vi "mainui.vi"() -> ()   [LabVIEW 2011]
uses:
  <vilib>/Platform/TimedLoop/XDataNode/timing_clust.ctl
  <vilib>/Platform/TimedLoop/XDataNode/nitl_modes.ctl
  <vilib>/Platform/TimedLoop/XDataNode/wakeup.ctl
  <vilib>/Utility/config.llb/Read Key (Double).vi
  <vilib>/Utility/config.llb/Read Key (I32).vi
  <vilib>/Utility/config.llb/Read Key (String).vi
  <vilib>/Utility/config.llb/Write Key (Double).vi
  <vilib>/Utility/config.llb/Write Key (I32).vi
  <vilib>/Utility/config.llb/Write Key (String).vi
  <vilib>/Platform/TimedLoop/XDataNode/XDataNode.xnode
  API/API DYM.lvlib
  <vilib>/Platform/TimedLoop/XDataNode/XDNodeRunTimeDep.lvlib
  <vilib>/Utility/config.llb/NI_LVConfig.lvlib
panel:
  in  "选项卡控件Next":enum32{"选项卡 1", "选项卡 2"}(tab)
  in  "BaseBtn":bool
  in  "MotinAdv":bool
  in  "restartbtn":bool
  in  "No1Btn":bool
  in  "No2Btn":bool
  in  "No3Btn":bool
  in  "Sensor":bool
  in  "选项卡控件":T1(tab)
  in  "ClearButton":bool
  out "红外计数":dbl
  out "电涡流计数":dbl
  out "红外电平":dbl
  out "电涡流电平":dbl
  out "电容1":dbl
  out "电容2":dbl
  out "电容3":dbl
  out "电桥电平":dbl
  out "电桥称重":dbl
  out "Waveform Chart":dynamicdata(graph)
  out "M1":bool
  out "M2":bool
  out "M3":bool
  out "M4":bool
  out "M5":bool
  out "M6":bool
  out "Plat3IO1":bool
  out "Plat3IO2":bool
  out "Plat3IO3":bool
  out "Plat3IO4":bool
  out "Plat3IO5":bool
  out "Plat3IO6":bool
  out "Plat3IO7":bool
  out "Plat3IO8":bool
  out "Plat2IO1":bool
  out "Plat2IO2":bool
  out "Plat2IO3":bool
  out "Plat2IO4":bool
  out "Plat2IO5":bool
  out "Plat2IO6":bool
  out "Plat2IO7":bool
  out "Plat2IO8":bool
  out "Solen48":bool
  out "Solen47":bool
  out "Solen46":bool
  out "Solen45":bool
  out "Solen44":bool
  out "Solen43":bool
  out "Solen42":bool
  out "Solen41":bool
  out "Solen40":bool
  out "Solen39":bool
  out "Solen38":bool
  out "Solen37":bool
  out "Solen36":bool
  out "Solen35":bool
  out "Solen34":bool
  out "Solen33":bool
  out "Solen32":bool
  out "Solen31":bool
  out "Solen30":bool
  out "Solen29":bool
  out "Solen28":bool
  out "Solen27":bool
  out "Solen26":bool
  out "Solen25":bool
  out "Solen24":bool
  out "Solen23":bool
  out "Solen22":bool
  out "Solen21":bool
  out "Solen20":bool
  out "Solen19":bool
  out "Solen18":bool
  out "Solen17":bool
  out "Solen16":bool
  out "Solen15":bool
  out "Solen14":bool
  out "Solen13":bool
  out "Solen12":bool
  out "Solen11":bool
  out "Solen10":bool
  out "Solen9":bool
  out "Solen8":bool
  out "Solen7":bool
  out "Solen6":bool
  out "Solen5":bool
  out "Solen4":bool
  out "Solen3":bool
  out "Solen2":bool
  out "Solen1":bool
  out "Plat1IO1":bool
  out "Plat1IO2":bool
  out "Plat1IO3":bool
  out "Plat1IO4":bool
  out "Plat1IO5":bool
  out "Plat1IO6":bool
  out "Plat1IO7":bool
  out "Plat1IO8":bool
  in  "MinSpeed":i32
  in  "MaxSpeed":i32
  in  "Horizontal4":i32
  in  "Horizontal3":i32
  in  "Horizontal2":i32
  in  "Horizontal1":i32
  in  "Vax4":i32
  in  "Vax3":i32
  in  "Vax2":i32
  in  "Vax1":i32
  in  "SaveParam":bool
  in  "CalcKB":bool
  out "BCalcd":dbl
  out "KCalcd":dbl
  out "Stog":dbl
  in  "Set2":bool
  in  "Set1":bool
  out "电桥电平_Event":dbl
  out "Volt2":dbl
  out "Volt1":dbl
  in  "X2":dbl
  in  "X1":dbl
  out "BCurrent":dbl
  out "KCurrent":dbl
  in  "SelectPolicy":enum32{"使用最短路径算法", "使用最短时间算法", "使用默认速度算法"}(radio)
  in  "ComboPolicy":string(combo)
  in  "ShowImg":bool
  in  "SaveConfigXZ":bool
  in  "SetReset":bool
  in  "MotorSpeed":i32=1
  in  "MotorSpeedNum":i32=1 min=1 max=6 step=1
  in  "SetMotorSpeed":bool
  out "Motor6Pos":i32
  out "Motor5Pos":i32
  out "Motor4Pos":i32
  out "Motor3Pos":i32
  out "Motor2Pos":i32
  out "Motor1Pos":i32
  in  "ClearPos6":bool
  in  "ClearPos5":bool
  in  "ClearPos4":bool
  in  "ClearPos3":bool
  in  "ClearPos2":bool
  in  "ClearPos1":bool
  in  "StopMotorNum":i32=1 min=1 max=6 step=1
  in  "StepNum":i32=1 min=1 max=20000 step=1
  in  "Directon":string(combo)
  in  "MotorNum":i32=1 min=1 max=6 step=1
  in  "SolenPlatStatue_Event":string(combo)
  in  "SolenPlat_Event":i32 min=0 max=2 step=1
  in  "SolenStatue_Event":string(combo)
  in  "SolenNum_Event":i32 min=0 max=47 step=1
  in  "MotorStop":bool
  in  "MotorStart":bool
  in  "FeedMotorStop":bool
  in  "FeedMotorStart":bool
  in  "SolenAdvance":bool
  in  "SolenAction":bool
  out "指令数":i32
  out "Statue":bool
  in  "start":bool
  in  "stop":bool
  in  "statuebtn":bool
  in  "no3btn":bool
  in  "no2btn":bool
  in  "no1btn":bool
  # "连接状态"
  # "待执行指令"
  # "红外计数"
  # "电涡流计数"
  # "电桥物体称重"
  # "红外传感器电平"
  # "电涡流传感器电平"
  # "电容式传感器1电平"
  # "电容式传感器2电平"
  # "电容式传感器3电平"
  # "电桥传感器电平"
  # "继电器状态"
  # "输入口状态"
  # "电机运行状态"
  # "单台控制策略——点位控制"
  # "单台控制策略——书写控制"
  # "当前电桥传感器矫正参数"
  # "g"
  # "K值"
  # "B值"
  # "当前传感器电压"
  # "mv"
  # "当前转换重量"
  # "电桥传感器参数标定"
  # "K值"
  # "B值"
  # "g"
  # "砝码重量1"
  # "对应电压"
  # "mv"
  # "砝码重量2"
  # "对应电压"
  # "g"
  # "mv"
  # "立体仓库坐标参数"
  # "第一行定位坐标Z轴"
  # "第一列定位坐标X轴"
  # "第二行定位坐标Z轴"
  # "第二列定位坐标X轴"
  # "第三行定位坐标Z轴"
  # "第三列定位坐标X轴"
  # "第四行定位坐标Z轴"
  # "第四列定位坐标X轴"
  # "电机参数"
  # "放置策略"
  # "电机最大速度"
  # "电机最小速度"
  # "策略选择"
  # "脉冲/S"
  # "脉冲/S"
  # "电机联动算法"
  # "继电器状态"
  # "继电器编号"
  # "继电器状态"
  # "平台编号"
  # "(进料电机运行)"
  # "电机速度"
  # "电机编号"
  # "脉冲/S"
  # "(进料电机停止)"
  # "电机编号"
  # "方向"
  # "步数"
  # "(1-20000)"
  # "电机编号"
  # "1号电机位置值:"
  # "4号电机位置值:"
  # "2号电机位置值:"
  # "5号电机位置值:"
  # "3号电机位置值:"
  # "6号电机位置值:"
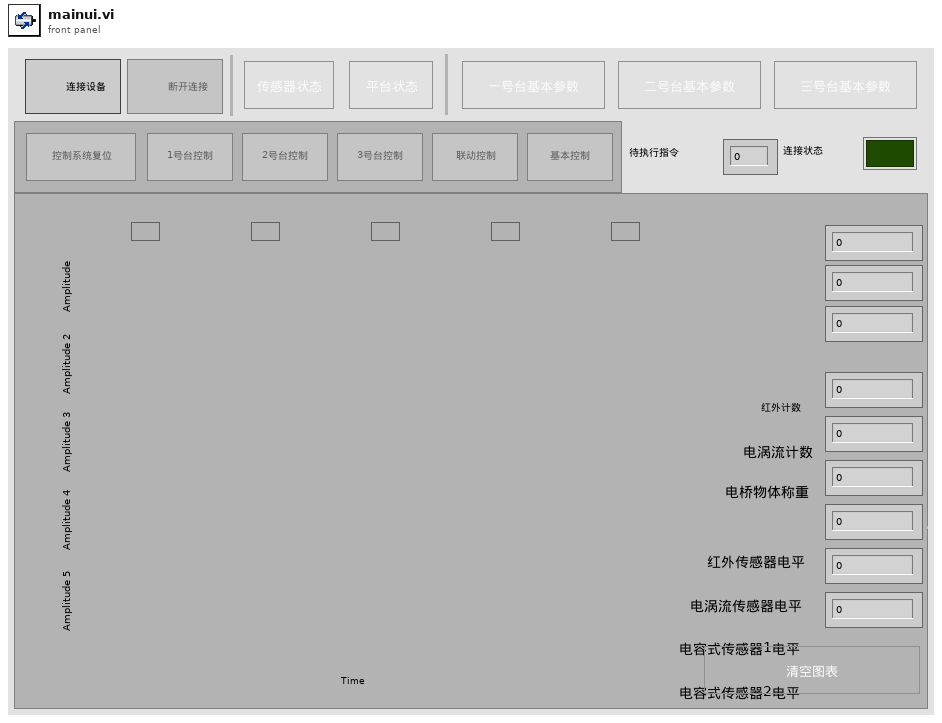
[diagram p1: front panel]
types:
  T1 = enum32{"选项卡 1", "选项卡 2", "选项卡 3", "选项卡 4", "选项卡 5", "选项卡 6"}
  T2 = enum8{"Enabled", "Disabled", "Disabled and Grayed Out"}
  T3 = enum16{"None", "GetSensorStatue", "GetSensorAD", "GetSolenStatue", "GetPaltformStatue", "GetMotorStatue", "FeedMotorStart", "FeedMotorStop", "MotorStart", "MotorRestart", "MotorStop", "SolenAction", "SolenAdv", "RcvDataInit", "SetMotorSpeed"}
  T4 = typedef "NI_LVConfig.lvlib/Config Data RefNum.ctl" = refnum<k1>
  T5 = enum16{"None", "GetSensorStatue", "GetSensorAD", "GetSolenStatue", "GetPaltformStatue", "GetMotorStatue", "FeedMotorStart", "FeedMotorStop", "MotorStart", "MotorRestart", "MotorStop", "SolenAction", "SolenAdv", "RcvDataInit"}
  T6 = typedef "XDNodeRunTimeDep.lvlib/timing_clust.ctl" = cluster{"Expected End [f-1]":u64, "Actual End [f-1]":u64, "Finished Late? [f-1]":bool, "Expected End [i-1]":u64, "Actual End [i-1]":u64, "Finished Late? [i-1]":bool, "Expected Start [i]":u64, "Actual Start [i]":u64, "Expected Start [f]":u64, "Actual Start [f]":u64, "Source Name":string, "Structure Name":string, "Period":i64, "Deadline":i64, "Offset":i64, "Start":i64, "Priority":i32, "Timeout":i32, "Mode":T7, "Wakeup Reason":T8, "Error":errorcluster, "Source Type":string, "Secondary Source Type":string, "Global End Time":u64, "Global Start Time":u64, "Frame Duration":u64, "Iteration Duration":u64, "Assigned CPU":i32, "I/O Scan Engine Mode":u32}
  T7 = typedef "XDNodeRunTimeDep.lvlib/nitl_modes.ctl" = enum32{"No Change", "Process missed periods, maintain original phase", "Discard missed periods, maintain original phase", "Process missed periods, ignore original phase", "Discard missed periods, ignore original phase"}
  T8 = typedef "XDNodeRunTimeDep.lvlib/wakeup.ctl" = enum32{"Normal", "Aborted", "Asynchronous wakeup", "Timing source error", "Timed loop error", "Timeout"}
  T9 = enum16{"None", "GetSensorStatue", "GetSensorAD", "GetSolenStatue", "GetPaltformStatue", "GetMotorStatue", "FeedMotorStart", "FeedMotorStop", "MotorStart", "MotorRestart", "MotorStop", "SolenAction", "SolenAdv"}
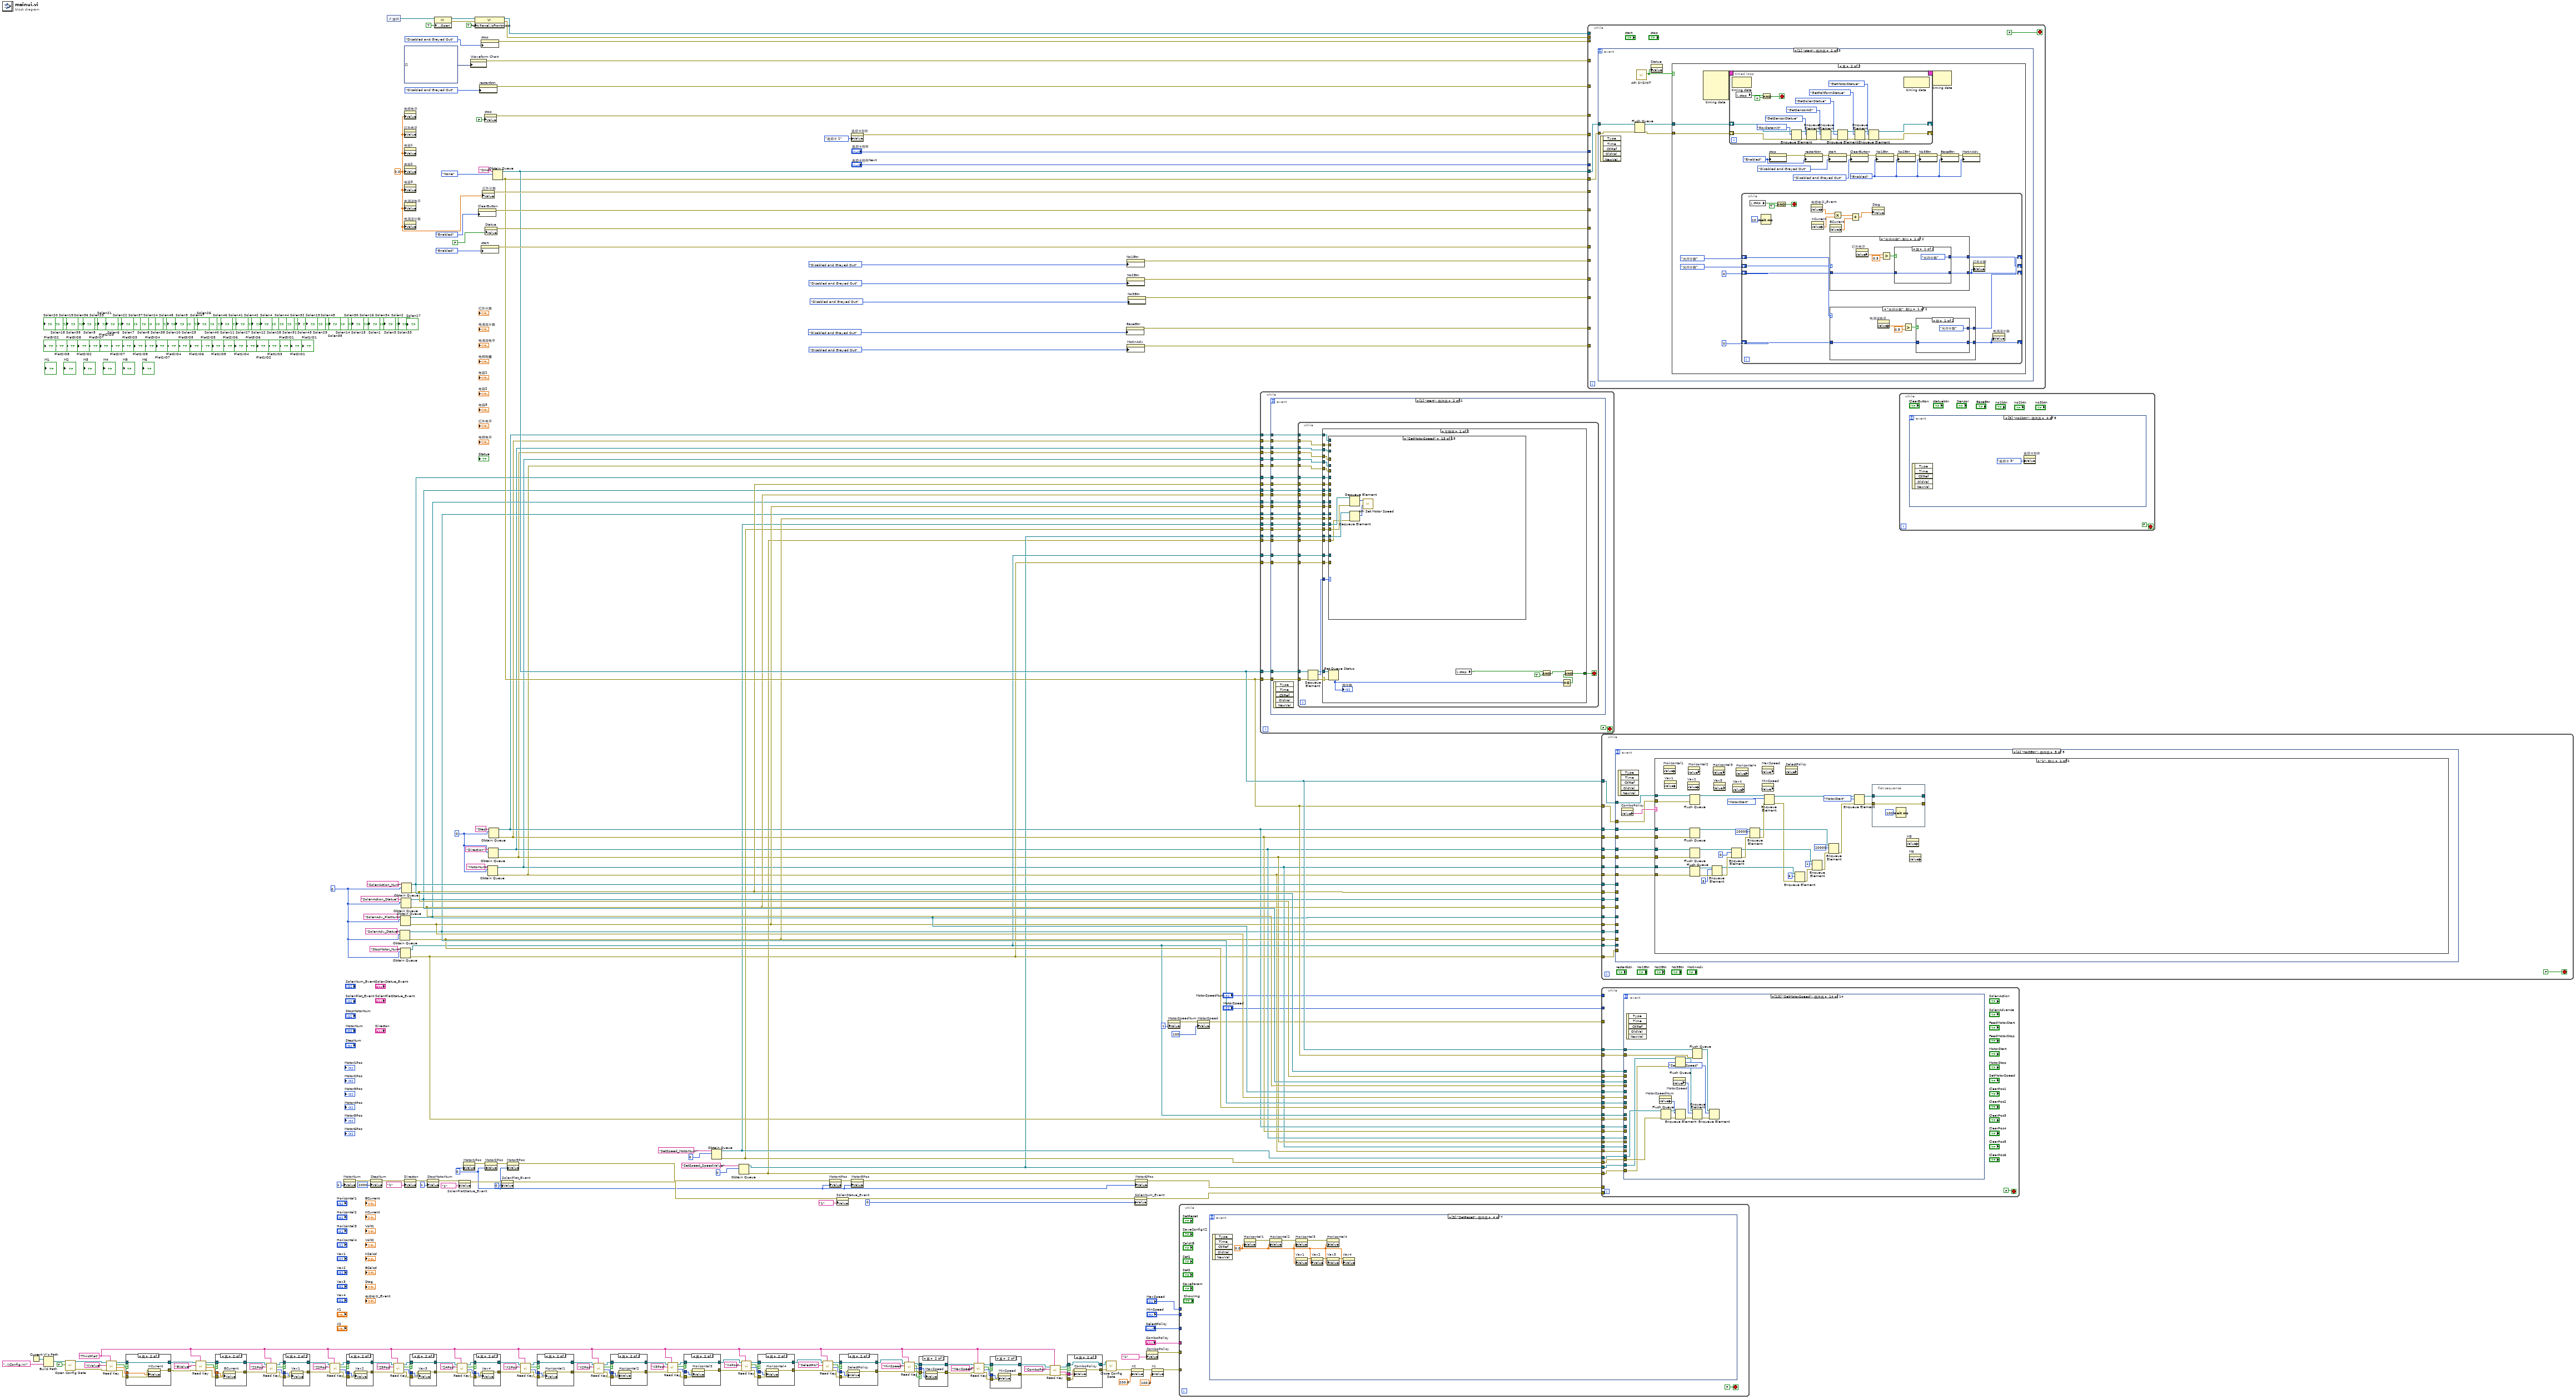
[diagram p0: block diagram]
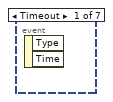
[diagram p16: hidden frame]
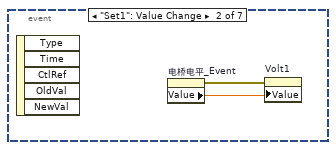
[diagram p17: hidden frame]
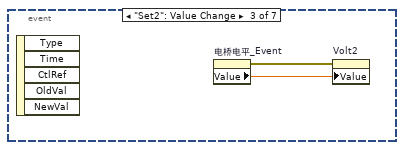
[diagram p18: hidden frame]
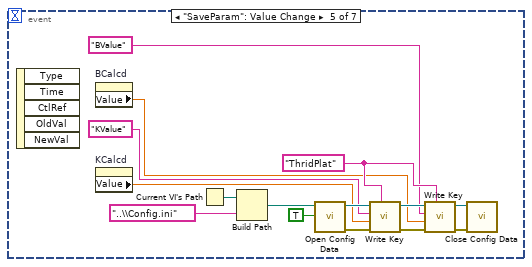
[diagram p19: hidden frame]
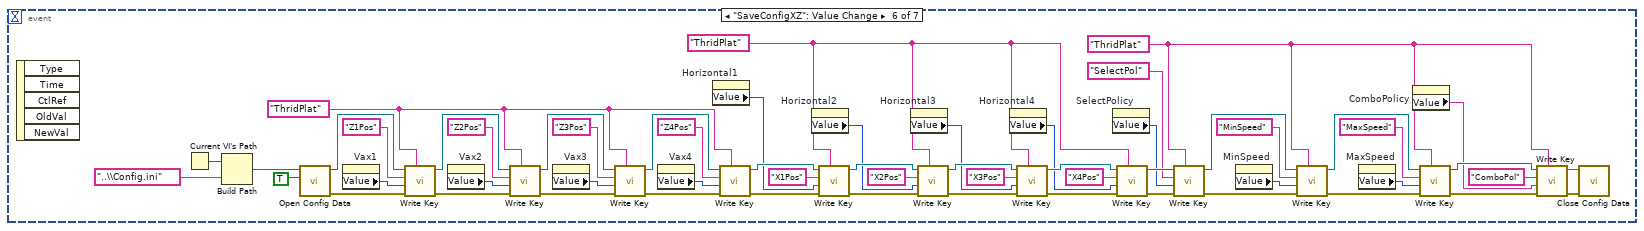
[diagram p20: hidden frame]
diagram:
  w2 = "ThridPlat" ("section")
  w135 = 0 ("Motor1Pos")
  w157 = 0
  w192 = 0
  w211 = 0.0
  n1 = Current VI's Path() -> (path=w129:path)
  n2 = Build Path(base path=w129, name or relative path="..\\Config.ini" ("名称或相对路径")) -> (appended path=w127:path)
  n3 = call <vilib>:"Open Config Data.vi"("create file if necessary (T)"=TRUE, "configuration file path"=w127) -> ("error out"=w124:errorcluster, "refnum"=w125:T4)  [unwired: 7 in, 1 out]
  n4 = call-poly <vilib>:"Read Key.vi"("section"=w2, "error in (no error)"=w124, "key"="KValue", "refnum"=w125) -> ("error out"=w120:errorcluster, "value"=w121:dbl, "found?"=w122:bool, "refnum out"=w119:T4)  [unwired: 4 in]
  n5 = case shown="真" w122 {
    tunnel: w121 -> [_ w226]
    tunnel: w120 -> [w221 w225]
    tunnel: [w221 w224] -> w117
    tunnel: [w222 w223] -> w118
    tunnel: w119 -> [w222 w223]
    frame False {
    }
    frame True {
      n6 = property on="KCurrent" class="DigNum (严格)"(error in=w225, "Value"=w226) -> (error out=w224:errorcluster)  [unwired: 1 in, 1 out]
    }
  }
  n7 = call-poly <vilib>:"Read Key.vi"("section"=w2, "error in (no error)"=w117, "key"="BValue", "refnum"=w118) -> ("error out"=w113:errorcluster, "value"=w112:dbl, "found?"=w115:bool, "refnum out"=w114:T4)  [unwired: 4 in]
  n8 = case shown="真" w115 {
    tunnel: [w228 w232] -> w111
    tunnel: w114 -> [w228 w232]
    tunnel: w113 -> [w227 w231]
    tunnel: [w227 w230] -> w110
    tunnel: w112 -> [_ w229]
    frame False {
    }
    frame True {
      n9 = property on="BCurrent" class="DigNum (严格)"(error in=w231, "Value"=w229) -> (error out=w230:errorcluster)  [unwired: 1 in, 1 out]
    }
  }
  n10 = call-poly <vilib>:"Read Key.vi"("section"=w2, "error in (no error)"=w110, "key"="Z1Pos", "refnum"=w111) -> ("error out"=w106:errorcluster, "value"=w105:i32, "found?"=w108:bool, "refnum out"=w107:T4)  [unwired: 4 in]
  n11 = case shown="真" w108 {
    tunnel: [w234 w238] -> w104
    tunnel: w107 -> [w234 w238]
    tunnel: w106 -> [w233 w237]
    tunnel: [w233 w236] -> w103
    tunnel: w105 -> [_ w235]
    frame False {
    }
    frame True {
      n12 = property on="Vax1" class="DigNum (严格)"(error in=w237, "Value"=w235) -> (error out=w236:errorcluster)  [unwired: 1 in, 1 out]
    }
  }
  n13 = call-poly <vilib>:"Read Key.vi"("section"=w2, "error in (no error)"=w103, "key"="Z2Pos", "refnum"=w104) -> ("error out"=w99:errorcluster, "value"=w98:i32, "found?"=w101:bool, "refnum out"=w100:T4)  [unwired: 4 in]
  n14 = property on="MotorNum" class="DigNum (严格)"("Value"=1 ("MotorNum")) -> (error out=w141:errorcluster)  [unwired: 2 in, 1 out]
  n15 = case shown="真" w101 {
    tunnel: w100 -> [w240 w244]
    tunnel: [w240 w244] -> w97
    tunnel: w99 -> [w239 w242]
    tunnel: w98 -> [_ w243]
    tunnel: [w239 w241] -> w96
    frame False {
    }
    frame True {
      n16 = property on="Vax2" class="DigNum (严格)"(error in=w242, "Value"=w243) -> (error out=w241:errorcluster)  [unwired: 1 in, 1 out]
    }
  }
  n17 = property on="StepNum" class="DigNum (严格)"(error in=w141, "Value"=2000 ("StepNum")) -> (error out=w144:errorcluster)  [unwired: 1 in, 1 out]
  n18 = control-ref of="本VI"() -> (w210:refnum<vi>)
  n19 = call-poly <vilib>:"Read Key.vi"("section"=w2, "error in (no error)"=w96, "key"="Z3Pos", "refnum"=w97) -> ("error out"=w92:errorcluster, "value"=w91:i32, "found?"=w94:bool, "refnum out"=w93:T4)  [unwired: 4 in]
  n20 = Obtain Queue(name (unnamed)="SolenAdv_Statue" ("名称（未命名）"), element data type=w157) -> (queue out=w160:refnum<queue>, error out=w159:errorcluster)  [unwired: 3 in, 1 out]
  n21 = Obtain Queue(name (unnamed)="SolenAdv_PlatNum" ("名称（未命名）"), element data type=w157) -> (queue out=w162:refnum<queue>, error out=w161:errorcluster)  [unwired: 3 in, 1 out]
  n22 = Obtain Queue(name (unnamed)="StopMotor_Num" ("名称（未命名）"), element data type=w157) -> (queue out=w156:refnum<queue>, error out=w155:errorcluster)  [unwired: 3 in, 1 out]
  n23 = Obtain Queue(name (unnamed)="SolenAction_Statue" ("名称（未命名）"), element data type=w157) -> (queue out=w168:refnum<queue>, error out=w167:errorcluster)  [unwired: 3 in, 1 out]
  n24 = Obtain Queue(name (unnamed)="SolenAction_Num" ("名称（未命名）"), element data type=w157) -> (queue out=w170:refnum<queue>, error out=w169:errorcluster)  [unwired: 3 in, 1 out]
  n25 = property on="电桥电平" class="DigNum (严格)"("Value"=w211) -> ()  [unwired: 2 in, 2 out]
  n26 = property on="红外电平" class="DigNum (严格)"("Value"=w211) -> ()  [unwired: 2 in, 2 out]
  n27 = property on="电容1" class="DigNum (严格)"("Value"=w211) -> ()  [unwired: 2 in, 2 out]
  n28 = property on="电容2" class="DigNum (严格)"("Value"=w211) -> ()  [unwired: 2 in, 2 out]
  n29 = property on="电容3" class="DigNum (严格)"("Value"=w211) -> ()  [unwired: 2 in, 2 out]
  n30 = property on="电涡流电平" class="DigNum (严格)"("Value"=w211) -> ()  [unwired: 2 in, 2 out]
  n31 = property on="电涡流计数" class="DigNum (严格)"("Value"=w211) -> ()  [unwired: 2 in, 2 out]
  n32 = property on="Directon" class="CmbBox"(error in=w144, "Value"="1" ("Directon")) -> (error out=w145:errorcluster)  [unwired: 1 in, 1 out]
  n33 = case shown="真" w94 {
    tunnel: w93 -> [w246 w250]
    tunnel: [w246 w250] -> w90
    tunnel: w92 -> [w245 w248]
    tunnel: w91 -> [_ w249]
    tunnel: [w245 w247] -> w89
    frame False {
    }
    frame True {
      n34 = property on="Vax3" class="DigNum (严格)"(error in=w248, "Value"=w249) -> (error out=w247:errorcluster)  [unwired: 1 in, 1 out]
    }
  }
  n35 = property on="StopMotorNum" class="DigNum (严格)"(error in=w145, "Value"=1 ("StopMotorNum")) -> (error out=w147:errorcluster)  [unwired: 1 in, 1 out]
  n36 = property class="VI"(reference=w210, "Front Panel.Open"=TRUE ("前面板窗口:打开")) -> (reference out=w208:refnum<vi>, error out=w207:errorcluster)  [unwired: 1 in]
  n37 = call-poly <vilib>:"Read Key.vi"("section"=w2, "error in (no error)"=w89, "key"="Z4Pos", "refnum"=w90) -> ("error out"=w85:errorcluster, "value"=w84:i32, "found?"=w87:bool, "refnum out"=w86:T4)  [unwired: 4 in]
  n38 = property on="SolenPlatStatue_Event" class="CmbBox"(error in=w147, "Value"="1" ("SolenPlatStatue_Event")) -> (error out=w164:errorcluster)  [unwired: 1 in, 1 out]
  n39 = property on="Motor1Pos" class="DigNum (严格)"("Value"=w135) -> (error out=w139:errorcluster)  [unwired: 2 in, 1 out]
  n40 = property on="Waveform Chart" class="WFChart (严格)"("History Data"=dynamicdata[] [] ("历史数据")) -> (error out=w218:errorcluster)  [unwired: 2 in, 1 out]
  n41 = case shown="真" w87 {
    tunnel: w86 -> [w252 w256]
    tunnel: w85 -> [w251 w254]
    tunnel: [w252 w256] -> w83
    tunnel: w84 -> [_ w255]
    tunnel: [w251 w253] -> w82
    frame False {
    }
    frame True {
      n42 = property on="Vax4" class="DigNum (严格)"(error in=w254, "Value"=w255) -> (error out=w253:errorcluster)  [unwired: 1 in, 1 out]
    }
  }
  n43 = property class="VI"(reference=w208, error in=w207, "Front Panel.IsFrontmost"=TRUE ("前面板窗口:在最前")) -> (reference out=w206:refnum<vi>, error out=w205:errorcluster)
  n44 = property on="ClearButton" class="Bool (严格)"("DisabledEnum"=T2."Enabled" ("禁用")) -> (error out=w216:errorcluster)  [unwired: 2 in, 1 out]
  n45 = property on="restartbtn" class="Bool"("DisabledEnum"=T2."Disabled and Grayed Out" ("禁用")) -> (error out=w200:errorcluster)  [unwired: 2 in, 1 out]
  n46 = property on="stop" class="Bool (严格)"("DisabledEnum"=T2."Disabled and Grayed Out" ("禁用")) -> (error out=w214:errorcluster)  [unwired: 2 in, 1 out]
  n47 = property on="start" class="Bool"("DisabledEnum"=T2."Enabled" ("禁用")) -> (error out=w215:errorcluster)  [unwired: 2 in, 1 out]
  n48 = property on="红外计数" class="DigNum (严格)"("Value"=w211) -> (error out=w220:errorcluster)  [unwired: 2 in, 1 out]
  n49 = property on="stop" class="Bool (严格)"("Value"=FALSE ("stop")) -> (error out=w196:errorcluster)  [unwired: 2 in, 1 out]
  n50 = property on="Statue" class="Bool (严格)"("Value"=FALSE ("Statue")) -> (error out=w202:errorcluster)  [unwired: 2 in, 1 out]
  n51 = property on="Motor2Pos" class="DigNum (严格)"(error in=w139, "Value"=w135) -> (error out=w140:errorcluster)  [unwired: 1 in, 1 out]
  n52 = Obtain Queue(name (unnamed)="MotorNum" ("名称（未命名）"), element data type=w192) -> (queue out=w150:refnum<queue>, error out=w149:errorcluster)  [unwired: 3 in, 1 out]
  n53 = Obtain Queue(name (unnamed)="Direction" ("名称（未命名）"), element data type=w192) -> (queue out=w152:refnum<queue>, error out=w151:errorcluster)  [unwired: 3 in, 1 out]
  n54 = Obtain Queue(name (unnamed)="Step" ("名称（未命名）"), element data type=w192) -> (queue out=w154:refnum<queue>, error out=w153:errorcluster)  [unwired: 3 in, 1 out]
  n55 = Obtain Queue(name (unnamed)="Cmd" ("名称（未命名）"), element data type=T3."None") -> (queue out=w172:refnum<queue>, error out=w171:errorcluster)  [unwired: 3 in, 1 out]
  n56 = property on="SolenPlat_Event" class="DigNum (严格)"(error in=w164, "Value"=0 ("SolenPlat_Event")) -> (error out=w166:errorcluster)  [unwired: 1 in, 1 out]
  n57 = property on="Motor3Pos" class="DigNum (严格)"(error in=w140, "Value"=w135) -> (error out=w138:errorcluster)  [unwired: 1 in, 1 out]
  n58 = call-poly <vilib>:"Read Key.vi"("section"=w2, "error in (no error)"=w82, "key"="X1Pos", "refnum"=w83) -> ("error out"=w79:errorcluster, "value"=w78:i32, "found?"=w77:bool, "refnum out"=w80:T4)  [unwired: 4 in]
  n59 = case shown="真" w77 {
    tunnel: w80 -> [w258 w262]
    tunnel: w79 -> [w257 w260]
    tunnel: [w258 w262] -> w76
    tunnel: w78 -> [_ w261]
    tunnel: [w257 w259] -> w75
    frame False {
    }
    frame True {
      n60 = property on="Horizontal1" class="DigNum (严格)"(error in=w260, "Value"=w261) -> (error out=w259:errorcluster)  [unwired: 1 in, 1 out]
    }
  }
  n61 = call-poly <vilib>:"Read Key.vi"("section"=w2, "error in (no error)"=w75, "key"="X2Pos", "refnum"=w76) -> ("error out"=w69:errorcluster, "value"=w68:i32, "found?"=w71:bool, "refnum out"=w70:T4)  [unwired: 4 in]
  n62 = case shown="真" w71 {
    tunnel: w70 -> [w264 w265]
    tunnel: w69 -> [w263 w267]
    tunnel: w68 -> [_ w268]
    tunnel: [w263 w266] -> w58
    tunnel: [w264 w265] -> w59
    frame False {
    }
    frame True {
      n63 = property on="Horizontal2" class="DigNum (严格)"(error in=w267, "Value"=w268) -> (error out=w266:errorcluster)  [unwired: 1 in, 1 out]
    }
  }
  n64 = call-poly <vilib>:"Read Key.vi"("section"=w2, "error in (no error)"=w58, "key"="X3Pos", "refnum"=w59) -> ("error out"=w64:errorcluster, "value"=w65:i32, "found?"=w67:bool, "refnum out"=w66:T4)  [unwired: 4 in]
  n65 = case shown="真" w67 {
    tunnel: w66 -> [w270 w272]
    tunnel: w65 -> [_ w274]
    tunnel: w64 -> [w269 w273]
    tunnel: [w270 w272] -> w57
    tunnel: [w269 w271] -> w56
    frame False {
    }
    frame True {
      n66 = property on="Horizontal3" class="DigNum (严格)"(error in=w273, "Value"=w274) -> (error out=w271:errorcluster)  [unwired: 1 in, 1 out]
    }
  }
  n67 = Obtain Queue(name (unnamed)="SetSpeed_MotorNum" ("名称（未命名）"), element data type=0) -> (queue out=w38:refnum<queue>, error out=w37:errorcluster)  [unwired: 3 in, 1 out]
  n68 = Obtain Queue(name (unnamed)="SetSpeed_SpeedValue" ("名称（未命名）"), element data type=0) -> (queue out=w36:refnum<queue>, error out=w35:errorcluster)  [unwired: 3 in, 1 out]
  n69 = call-poly <vilib>:"Read Key.vi"("section"=w2, "error in (no error)"=w56, "key"="X4Pos", "refnum"=w57) -> ("error out"=w61:errorcluster, "value"=w60:i32, "found?"=w63:bool, "refnum out"=w62:T4)  [unwired: 4 in]
  n70 = case shown="真" w63 {
    tunnel: w62 -> [w276 w280]
    tunnel: w61 -> [w275 w279]
    tunnel: w60 -> [_ w277]
    tunnel: [w276 w280] -> w33
    tunnel: [w275 w278] -> w32
    frame False {
    }
    frame True {
      n71 = property on="Horizontal4" class="DigNum (严格)"(error in=w279, "Value"=w277) -> (error out=w278:errorcluster)  [unwired: 1 in, 1 out]
    }
  }
  n72 = call-poly <vilib>:"Read Key.vi"("section"=w2, "error in (no error)"=w32, "key"="SelectPol", "refnum"=w33) -> ("error out"=w28:errorcluster, "value"=w27:i32, "found?"=w30:bool, "refnum out"=w29:T4)  [unwired: 4 in]
  n73 = property on="Motor4Pos" class="DigNum (严格)"(error in=w138, "Value"=w135) -> (error out=w137:errorcluster)  [unwired: 1 in, 1 out]
  n74 = property on="SolenStatue_Event" class="CmbBox"(error in=w166, "Value"="1" ("SolenStatue_Event")) -> (error out=w174:errorcluster)  [unwired: 1 in, 1 out]
  n75 = case shown="真" w30 {
    tunnel: w29 -> [w282 w286]
    tunnel: w28 -> [w281 w284]
    tunnel: w27 -> [_ w285]
    tunnel: [w282 w286] -> w26
    tunnel: [w281 w283] -> w25
    frame False {
    }
    frame True {
      n76 = property on="SelectPolicy" class="RadioBtnsControl (严格)"(error in=w284, "Value"=w285) -> (error out=w283:errorcluster)  [unwired: 1 in, 1 out]
    }
  }
  n77 = property on="选项卡控件" class="TabCtl (严格)"("Value"=T1."选项卡 1" ("选项卡控件")) -> (error out=w187:errorcluster)  [unwired: 2 in, 1 out]
  n78 = property on="Motor5Pos" class="DigNum (严格)"(error in=w137, "Value"=w135) -> (error out=w136:errorcluster)  [unwired: 1 in, 1 out]
  n79 = call-poly <vilib>:"Read Key.vi"("section"=w2, "error in (no error)"=w25, "key"="MinSpeed", "refnum"=w26) -> ("error out"=w23:errorcluster, "value"=w21:i32, "found?"=w1:bool, "refnum out"=w24:T4)  [unwired: 4 in]
  n80 = case shown="真" w1 {
    tunnel: w24 -> [w288 w292]
    tunnel: [w288 w292] -> w20
    tunnel: w23 -> [w287 w290]
    tunnel: w21 -> [_ w291]
    tunnel: [w287 w289] -> w19
    frame False {
    }
    frame True {
      n81 = property on="MaxSpeed" class="DigNum (严格)"(error in=w290, "Value"=w291) -> (error out=w289:errorcluster)  [unwired: 1 in, 1 out]
    }
  }
  n82 = call-poly <vilib>:"Read Key.vi"("section"=w2, "error in (no error)"=w19, "key"="MaxSpeed", "refnum"=w20) -> ("error out"=w15:errorcluster, "value"=w14:i32, "found?"=w17:bool, "refnum out"=w16:T4)  [unwired: 4 in]
  n83 = case shown="真" w17 {
    tunnel: w16 -> [w294 w295]
    tunnel: w15 -> [w293 w298]
    tunnel: w14 -> [_ w297]
    tunnel: [w293 w296] -> w12
    tunnel: [w294 w295] -> w13
    frame False {
    }
    frame True {
      n84 = property on="MinSpeed" class="DigNum (严格)"(error in=w298, "Value"=w297) -> (error out=w296:errorcluster)  [unwired: 1 in, 1 out]
    }
  }
  n85 = call-poly <vilib>:"Read Key.vi"("section"=w2, "error in (no error)"=w12, "key"="ComboPol", "refnum"=w13) -> ("error out"=w9:errorcluster, "value"=w7:string, "found?"=w8:bool, "refnum out"=w10:T4)  [unwired: 4 in]
  n86 = case shown="真" w8 {
    tunnel: w10 -> [w300 w301]
    tunnel: w9 -> [w299 w303]
    tunnel: w7 -> [_ w304]
    tunnel: [w299 w302] -> w5
    tunnel: [w300 w301] -> w6
    frame False {
    }
    frame True {
      n87 = property on="ComboPolicy" class="CmbBox"(error in=w303, "Value"=w304) -> (error out=w302:errorcluster)  [unwired: 1 in, 1 out]
    }
  }
  n88 = call <vilib>:"Close Config Data.vi"("error in (no error)"=w5, "refnum"=w6) -> ("error out"=w55:errorcluster)  [unwired: 8 in, 1 out]
  n89 = property on="BaseBtn" class="Bool"("DisabledEnum"=T2."Disabled and Grayed Out" ("禁用")) -> (error out=w180:errorcluster)  [unwired: 2 in, 1 out]
  n90 = property on="No1Btn" class="Bool"("DisabledEnum"=T2."Disabled and Grayed Out" ("禁用")) -> (error out=w186:errorcluster)  [unwired: 2 in, 1 out]
  n91 = property on="No2Btn" class="Bool"("DisabledEnum"=T2."Disabled and Grayed Out" ("禁用")) -> (error out=w184:errorcluster)  [unwired: 2 in, 1 out]
  n92 = property on="MotinAdv" class="Bool"("DisabledEnum"=T2."Disabled and Grayed Out" ("禁用")) -> (error out=w178:errorcluster)  [unwired: 2 in, 1 out]
  n93 = property on="No3Btn" class="Bool"("DisabledEnum"=T2."Disabled and Grayed Out" ("禁用")) -> (error out=w183:errorcluster)  [unwired: 2 in, 1 out]
  n94 = property on="X2" class="DigNum (严格)"(error in=w55, "Value"=200.0 ("X2")) -> (error out=w130:errorcluster)  [unwired: 1 in, 1 out]
  n95 = property on="SolenNum_Event" class="DigNum (严格)"(error in=w174, "Value"=0 ("SolenNum_Event")) -> (error out=w176:errorcluster)  [unwired: 1 in, 1 out]
  n96 = property on="Motor6Pos" class="DigNum (严格)"(error in=w136, "Value"=w135) -> (error out=w134:errorcluster)  [unwired: 1 in, 1 out]
  n97 = property on="ComboPolicy" class="CmbBox"("Value"="1" ("ComboPolicy")) -> (error out=w34:errorcluster)  [unwired: 2 in, 1 out]
  n98 = property on="X1" class="DigNum (严格)"(error in=w130, "Value"=100.0 ("X1")) -> (error out=w132:errorcluster)  [unwired: 1 in, 1 out]
  n99 = property on="MotorSpeedNum" class="DigNum (严格)"("Value"=1 ("MotorSpeedNum")) -> (error out=w48:errorcluster)  [unwired: 2 in, 1 out]
  n100 = while {
    tunnel: w132 -> [_]
    tunnel: "SelectPolicy" -> [_]
    tunnel: "ComboPolicy" -> [_]
    tunnel: "MaxSpeed" -> [_]
    tunnel: "MinSpeed" -> [_]
    tunnel: w34 -> [_]
    stop <- FALSE stop-if-true
    n101 = event shown="[3] \"SetReset\": 值改变" {
      selector: _ -> [_ _ _ _ _ _ _]
      dyn-events: _ -> [_ _ _ _ _ _ _]
      timeout: _ -> [_ _ _ _ _ _ _]
      event Timeout {
        n102 = event-data() -> ()  [unwired: 1 in, 2 out]
      }
      event "Set1": Value Change {
        n103 = event-data() -> ()  [unwired: 1 in, 5 out]
        n104 = property on="电桥电平_Event" class="DigNum (严格)"() -> (error out=w306:errorcluster, "Value"=w307:dbl)  [unwired: 2 in, 1 out]
        n105 = property on="Volt1" class="DigNum (严格)"(error in=w306, "Value"=w307) -> ()  [unwired: 1 in, 2 out]
      }
      event "Set2": Value Change {
        n106 = event-data() -> ()  [unwired: 1 in, 5 out]
        n107 = property on="电桥电平_Event" class="DigNum (严格)"() -> (error out=w309:errorcluster, "Value"=w308:dbl)  [unwired: 2 in, 1 out]
        n108 = property on="Volt2" class="DigNum (严格)"(error in=w309, "Value"=w308) -> ()  [unwired: 1 in, 2 out]
      }
      event "SetReset": Value Change {
        w310 = 0.0 ("Horizontal1")
        n109 = event-data() -> ()  [unwired: 1 in, 5 out]
        n110 = property on="Horizontal1" class="DigNum (严格)"("Value"=w310) -> (error out=w316:errorcluster)  [unwired: 2 in, 1 out]
        n111 = property on="Horizontal2" class="DigNum (严格)"(error in=w316, "Value"=w310) -> (error out=w315:errorcluster)  [unwired: 1 in, 1 out]
        n112 = property on="Horizontal3" class="DigNum (严格)"(error in=w315, "Value"=w310) -> (error out=w314:errorcluster)  [unwired: 1 in, 1 out]
        n113 = property on="Vax1" class="DigNum (严格)"("Value"=w310) -> (error out=w313:errorcluster)  [unwired: 2 in, 1 out]
        n114 = property on="Vax2" class="DigNum (严格)"(error in=w313, "Value"=w310) -> (error out=w312:errorcluster)  [unwired: 1 in, 1 out]
        n115 = property on="Horizontal4" class="DigNum (严格)"(error in=w314, "Value"=w310) -> ()  [unwired: 1 in, 2 out]
        n116 = property on="Vax3" class="DigNum (严格)"(error in=w312, "Value"=w310) -> (error out=w311:errorcluster)  [unwired: 1 in, 1 out]
        n117 = property on="Vax4" class="DigNum (严格)"(error in=w311, "Value"=w310) -> ()  [unwired: 1 in, 2 out]
      }
      event "SaveParam": Value Change {
        w323 = "ThridPlat" ("section")
        n118 = event-data() -> ()  [unwired: 1 in, 5 out]
        n119 = property on="BCalcd" class="DigNum (严格)"() -> ("Value"=w319:dbl)  [unwired: 2 in, 2 out]
        n120 = property on="KCalcd" class="DigNum (严格)"() -> ("Value"=w320:dbl)  [unwired: 2 in, 2 out]
        n121 = Current VI's Path() -> (path=w331:path)
        n122 = Build Path(base path=w331, name or relative path="..\\Config.ini" ("名称或相对路径")) -> (appended path=w329:path)
        n123 = call <vilib>:"Open Config Data.vi"("create file if necessary (T)"=TRUE, "configuration file path"=w329) -> ("error out"=w326:errorcluster, "refnum"=w327:T4)  [unwired: 7 in, 1 out]
        n124 = call-poly <vilib>:"Write Key.vi"("section"=w323, "error in (no error)"=w326, "value"=w320, "key"="KValue", "refnum"=w327) -> ("error out"=w324:errorcluster, "refnum out"=w325:T4)  [unwired: 4 in, 1 out]
        n125 = call-poly <vilib>:"Write Key.vi"("section"=w323, "error in (no error)"=w324, "value"=w319, "key"="BValue", "refnum"=w325) -> ("error out"=w317:errorcluster, "refnum out"=w318:T4)  [unwired: 4 in, 1 out]
        n126 = call <vilib>:"Close Config Data.vi"("error in (no error)"=w317, "refnum"=w318) -> ()  [unwired: 8 in, 2 out]
      }
      event "SaveConfigXZ": Value Change {
        w340 = "ThridPlat" ("section")
        w369 = "ThridPlat" ("section")
        w370 = "ThridPlat" ("section")
        n127 = event-data() -> ()  [unwired: 1 in, 5 out]
        n128 = Current VI's Path() -> (path=w388:path)
        n129 = Build Path(base path=w388, name or relative path="..\\Config.ini" ("名称或相对路径")) -> (appended path=w386:path)
        n130 = call <vilib>:"Open Config Data.vi"("create file if necessary (T)"=TRUE, "configuration file path"=w386) -> ("error out"=w365:errorcluster, "refnum"=w384:T4)  [unwired: 7 in, 1 out]
        n131 = property on="Vax1" class="DigNum (严格)"() -> ("Value"=w382:i32)  [unwired: 2 in, 2 out]
        n132 = call-poly <vilib>:"Write Key.vi"("section"=w370, "error in (no error)"=w365, "value"=w382, "key"="Z1Pos", "refnum"=w384) -> ("error out"=w378:errorcluster, "refnum out"=w381:T4)  [unwired: 4 in, 1 out]
        n133 = property on="Vax2" class="DigNum (严格)"() -> ("Value"=w358:i32)  [unwired: 2 in, 2 out]
        n134 = call-poly <vilib>:"Write Key.vi"("section"=w370, "error in (no error)"=w378, "value"=w358, "key"="Z2Pos", "refnum"=w381) -> ("error out"=w377:errorcluster, "refnum out"=w380:T4)  [unwired: 4 in, 1 out]
        n135 = property on="Vax3" class="DigNum (严格)"() -> ("Value"=w357:i32)  [unwired: 2 in, 2 out]
        n136 = call-poly <vilib>:"Write Key.vi"("section"=w370, "error in (no error)"=w377, "value"=w357, "key"="Z3Pos", "refnum"=w380) -> ("error out"=w376:errorcluster, "refnum out"=w379:T4)  [unwired: 4 in, 1 out]
        n137 = property on="Vax4" class="DigNum (严格)"() -> ("Value"=w355:i32)  [unwired: 2 in, 2 out]
        n138 = property on="Horizontal1" class="DigNum (严格)"() -> ("Value"=w354:i32)  [unwired: 2 in, 2 out]
        n139 = call-poly <vilib>:"Write Key.vi"("section"=w370, "error in (no error)"=w376, "value"=w355, "key"="Z4Pos", "refnum"=w379) -> ("error out"=w371:errorcluster, "refnum out"=w372:T4)  [unwired: 4 in, 1 out]
        n140 = property on="Horizontal2" class="DigNum (严格)"() -> ("Value"=w353:i32)  [unwired: 2 in, 2 out]
        n141 = call-poly <vilib>:"Write Key.vi"("section"=w369, "error in (no error)"=w371, "value"=w354, "key"="X1Pos", "refnum"=w372) -> ("error out"=w373:errorcluster, "refnum out"=w368:T4)  [unwired: 4 in, 1 out]
        n142 = property on="Horizontal3" class="DigNum (严格)"() -> ("Value"=w352:i32)  [unwired: 2 in, 2 out]
        n143 = call-poly <vilib>:"Write Key.vi"("section"=w369, "error in (no error)"=w373, "value"=w353, "key"="X2Pos", "refnum"=w368) -> ("error out"=w374:errorcluster, "refnum out"=w367:T4)  [unwired: 4 in, 1 out]
        n144 = property on="Horizontal4" class="DigNum (严格)"() -> ("Value"=w351:i32)  [unwired: 2 in, 2 out]
        n145 = call-poly <vilib>:"Write Key.vi"("section"=w369, "error in (no error)"=w374, "value"=w352, "key"="X3Pos", "refnum"=w367) -> ("error out"=w375:errorcluster, "refnum out"=w366:T4)  [unwired: 4 in, 1 out]
        n146 = property on="SelectPolicy" class="RadioBtnsControl (严格)"() -> ("Value"=w335:enum32{"使用最短路径算法", "使用最短时间算法", "使用默认速度算法"})  [unwired: 2 in, 2 out]
        n147 = call-poly <vilib>:"Write Key.vi"("section"=w369, "error in (no error)"=w375, "value"=w351, "key"="X4Pos", "refnum"=w366) -> ("error out"=w349:errorcluster, "refnum out"=w350:T4)  [unwired: 4 in, 1 out]
        n148 = call-poly <vilib>:"Write Key.vi"("section"=w340, "error in (no error)"=w349, "value"=w335, "key"="SelectPol", "refnum"=w350) -> ("error out"=w347:errorcluster, "refnum out"=w348:T4)  [unwired: 4 in, 1 out]
        n149 = property on="MinSpeed" class="DigNum (严格)"() -> ("Value"=w334:i32)  [unwired: 2 in, 2 out]
        n150 = call-poly <vilib>:"Write Key.vi"("section"=w340, "error in (no error)"=w347, "value"=w334, "key"="MinSpeed", "refnum"=w348) -> ("error out"=w345:errorcluster, "refnum out"=w346:T4)  [unwired: 4 in, 1 out]
        n151 = property on="MaxSpeed" class="DigNum (严格)"() -> ("Value"=w333:i32)  [unwired: 2 in, 2 out]
        n152 = property on="ComboPolicy" class="CmbBox"() -> ("Value"=w332:string)  [unwired: 2 in, 2 out]
        n153 = call-poly <vilib>:"Write Key.vi"("section"=w340, "error in (no error)"=w345, "value"=w333, "key"="MaxSpeed", "refnum"=w346) -> ("error out"=w343:errorcluster, "refnum out"=w344:T4)  [unwired: 4 in, 1 out]
        n154 = call-poly <vilib>:"Write Key.vi"("section"=w340, "error in (no error)"=w343, "value"=w332, "key"="ComboPol", "refnum"=w344) -> ("error out"=w341:errorcluster, "refnum out"=w342:T4)  [unwired: 4 in, 1 out]
        n155 = call <vilib>:"Close Config Data.vi"("error in (no error)"=w341, "refnum"=w342) -> ()  [unwired: 8 in, 2 out]
      }
      event "CalcKB": Value Change {
        n156 = event-data() -> ()  [unwired: 1 in, 5 out]
        n157 = property on="Volt1" class="DigNum (严格)"() -> ("Value"=w390:dbl)  [unwired: 2 in, 2 out]
        n158 = property on="Volt2" class="DigNum (严格)"() -> ("Value"=w389:dbl)  [unwired: 2 in, 2 out]
        n159 = Not Equal?(x=w390, y=w389) -> (x != y?=w391:bool)
        n160 = case shown="假" w391 {
          tunnel: w390 -> [_ w401]
          tunnel: w389 -> [_ w396]
          frame False {
            n161 = One Button Dialog(message="计算发生错误 !" ("消息")) -> ()  [unwired: 1 in, 1 out]
          }
          frame True {
            n162 = property on="X2" class="DigNum (严格)"() -> ("Value"=w394:dbl)  [unwired: 2 in, 2 out]
            n163 = property on="X1" class="DigNum (严格)"() -> ("Value"=w400:dbl)  [unwired: 2 in, 2 out]
            n164 = Subtract(x=w401, y=w396) -> (x-y=w398:dbl)
            n165 = Subtract(x=w400, y=w394) -> (x-y=w399:dbl)
            n166 = Divide(x=w399, y=w398) -> (x/y=w397:dbl)
            n167 = Multiply(x=w397, y=w396) -> (x*y=w395:dbl)
            n168 = Subtract(x=w394, y=w395) -> (x-y=w393:dbl)
            n169 = property on="KCalcd" class="DigNum (严格)"("Value"=w397) -> ()  [unwired: 2 in, 2 out]
            n170 = property on="BCalcd" class="DigNum (严格)"("Value"=w393) -> ()  [unwired: 2 in, 2 out]
          }
        }
      }
    }
  }
  n171 = property on="MotorSpeed" class="DigNum (严格)"(error in=w48, "Value"=100 ("MotorSpeed")) -> (error out=w47:errorcluster)  [unwired: 1 in, 1 out]
  n172 = while {
    tunnel: w172 -> [w422]
    tunnel: w171 -> [w423]
    tunnel: w154 -> [w421]
    tunnel: w153 -> [w420]
    tunnel: w152 -> [w419]
    tunnel: w151 -> [w418]
    tunnel: w150 -> [w417]
    tunnel: w149 -> [w416]
    tunnel: w170 -> [w415]
    tunnel: w169 -> [w414]
    tunnel: w168 -> [w413]
    tunnel: w167 -> [w412]
    tunnel: w162 -> [w411]
    tunnel: w161 -> [w410]
    tunnel: w160 -> [w409]
    tunnel: w159 -> [w408]
    tunnel: w156 -> [w407]
    tunnel: w155 -> [w406]
    tunnel: w38 -> [w405]
    tunnel: w37 -> [w404]
    tunnel: w36 -> [w403]
    tunnel: w35 -> [w402]
    stop <- FALSE stop-if-true
    n173 = event shown="[1] \"start\": 值改变" {
      selector: _ -> [_ _]
      dyn-events: _ -> [_ _]
      timeout: _ -> [_ _]
      tunnel: w423 -> [_ w446]
      tunnel: w422 -> [_ w445]
      tunnel: w421 -> [_ w444]
      tunnel: w420 -> [_ w443]
      tunnel: w419 -> [_ w442]
      tunnel: w418 -> [_ w441]
      tunnel: w417 -> [_ w440]
      tunnel: w416 -> [_ w439]
      tunnel: w415 -> [_ w438]
      tunnel: w414 -> [_ w437]
      tunnel: w413 -> [_ w436]
      tunnel: w412 -> [_ w435]
      tunnel: w411 -> [_ w434]
      tunnel: w410 -> [_ w433]
      tunnel: w409 -> [_ w432]
      tunnel: w408 -> [_ w431]
      tunnel: w407 -> [_ w430]
      tunnel: w406 -> [_ w429]
      tunnel: w405 -> [_ w428]
      tunnel: w404 -> [_ w427]
      tunnel: w403 -> [_ w426]
      tunnel: w402 -> [_ w425]
      event Timeout {
        n174 = event-data() -> ()  [unwired: 1 in, 2 out]
      }
      event "start": Value Change {
        n175 = event-data() -> ()  [unwired: 1 in, 5 out]
        n176 = while {
          tunnel: w446 -> [w467]
          tunnel: w445 -> [w468]
          tunnel: w444 -> [w462]
          tunnel: w443 -> [w461]
          tunnel: w442 -> [w464]
          tunnel: w441 -> [w463]
          tunnel: w440 -> [w466]
          tunnel: w439 -> [w465]
          tunnel: w438 -> [w460]
          tunnel: w437 -> [w459]
          tunnel: w436 -> [w458]
          tunnel: w435 -> [w457]
          tunnel: w434 -> [w456]
          tunnel: w433 -> [w455]
          tunnel: w432 -> [w454]
          tunnel: w431 -> [w453]
          tunnel: w430 -> [w452]
          tunnel: w429 -> [w451]
          tunnel: w428 -> [w450]
          tunnel: w427 -> [w449]
          tunnel: w426 -> [w448]
          tunnel: w425 -> [w447]
          stop <- w471 stop-if-true
          n177 = Dequeue Element(queue=w468, error in (no error)=w467) -> (queue out=w469:refnum<queue>, element=w472:T3, error out=w470:errorcluster)  [unwired: 1 in, 1 out]
          n178 = case shown="无错误" w470 {
            selector: w470 -> [w499 _]
            tunnel: w472 -> [w501 _]
            tunnel: [w479 TRUE] -> w471
            tunnel: w469 -> [w500 _]
            tunnel: w466 -> [w496 _]
            tunnel: w465 -> [w495 _]
            tunnel: w464 -> [w494 _]
            tunnel: w463 -> [w493 _]
            tunnel: w462 -> [w492 _]
            tunnel: w461 -> [w491 _]
            tunnel: w460 -> [w490 _]
            tunnel: w459 -> [w489 _]
            tunnel: w458 -> [w488 _]
            tunnel: w457 -> [w487 _]
            tunnel: w456 -> [w486 _]
            tunnel: w455 -> [w485 _]
            tunnel: w454 -> [w484 _]
            tunnel: w453 -> [w483 _]
            tunnel: w452 -> [w478 _]
            tunnel: w451 -> [w477 _]
            tunnel: w450 -> [w476 _]
            tunnel: w449 -> [w474 _]
            tunnel: w448 -> [w475 _]
            tunnel: w447 -> [w473 _]
            frame No Error {
              n179 = case shown="\"SetMotorSpeed\"" w501 {
                tunnel: w496 -> [_ _ _ _ _ _ _ _ w594 _ _ _ _ _ _]
                tunnel: w495 -> [_ _ _ _ _ _ _ _ w593 _ _ _ _ _ _]
                tunnel: w494 -> [_ _ _ _ _ _ _ _ w597 _ _ _ _ _ _]
                tunnel: w493 -> [_ _ _ _ _ _ _ _ w596 _ _ _ _ _ _]
                tunnel: w492 -> [_ _ _ _ _ _ _ _ w600 _ _ _ _ _ _]
                tunnel: w491 -> [_ _ _ _ _ _ _ _ w599 _ _ _ _ _ _]
                tunnel: w490 -> [_ _ _ _ _ _ _ _ _ _ _ w606 _ _ _]
                tunnel: w489 -> [_ _ _ _ _ _ _ _ _ _ _ w605 _ _ _]
                tunnel: w488 -> [_ _ _ _ _ _ _ _ _ _ _ w604 _ _ _]
                tunnel: w487 -> [_ _ _ _ _ _ _ _ _ _ _ w603 _ _ _]
                tunnel: w486 -> [_ _ _ _ _ _ _ _ _ _ _ _ w612 _ _]
                tunnel: w485 -> [_ _ _ _ _ _ _ _ _ _ _ _ w611 _ _]
                tunnel: w484 -> [_ _ _ _ _ _ _ _ _ _ _ _ w610 _ _]
                tunnel: w483 -> [_ _ _ _ _ _ _ _ _ _ _ _ w609 _ _]
                tunnel: w478 -> [_ _ _ _ _ _ _ _ _ _ _ _ _ _ _]
                tunnel: w477 -> [_ _ _ _ _ _ _ _ _ _ _ _ _ _ _]
                tunnel: w476 -> [_ _ _ _ _ _ _ _ _ _ _ _ _ _ w618]
                tunnel: w475 -> [_ _ _ _ _ _ _ _ _ _ _ _ _ _ w616]
                tunnel: w474 -> [_ _ _ _ _ _ _ _ _ _ _ _ _ _ w617]
                tunnel: w473 -> [_ _ _ _ _ _ _ _ _ _ _ _ _ _ w615]
                frame "None", Default {
                }
                frame "GetSensorStatue" {
                  n180 = Initialize Array(0 ("元素"), 8 ("维数大小")) -> (w504:i32[])
                  n181 = call "API get Sensor Statue.vi"("array input"=w504) -> ("array output"=w510:i32[])  [unwired: 9 in, 1 out]
                  n182 = Index Array(array=w510, index=2 ("索引")) -> (element=w518:i32)
                  n183 = Index Array(array=w510, index=1 ("索引")) -> (element=w517:i32)
                  n184 = Index Array(array=w510, index=4 ("索引")) -> (element=w519:i32)
                  n185 = Index Array(array=w510, index=5 ("索引")) -> (element=w520:i32)
                  n186 = Index Array(array=w510, index=3 ("索引")) -> (element=w521:i32)
                  n187 = property on="红外电平" class="DigNum (严格)"("Value"=w518) -> ()  [unwired: 2 in, 2 out]
                  n188 = property on="电涡流电平" class="DigNum (严格)"("Value"=w517) -> ()  [unwired: 2 in, 2 out]
                  n189 = property on="电容1" class="DigNum (严格)"("Value"=w519) -> ()  [unwired: 2 in, 2 out]
                  n190 = property on="电容2" class="DigNum (严格)"("Value"=w520) -> ()  [unwired: 2 in, 2 out]
                  n191 = property on="电容3" class="DigNum (严格)"("Value"=w521) -> ()  [unwired: 2 in, 2 out]
                  n192 = Merge Signals(w518) -> (w515:dynamicdata)
                  n193 = Merge Signals(w517) -> (w516:dynamicdata)
                  n194 = Merge Signals(w519) -> (w511:dynamicdata)
                  n195 = Merge Signals(w520) -> (w513:dynamicdata)
                  n196 = Merge Signals(w521) -> (w512:dynamicdata)
                  n197 = Merge Signals(w515, w516, w511, w513, w512) -> (→"Waveform Chart":dynamicdata)
                }
                frame "GetSensorAD" {
                  n198 = call "API get Sensor AD.vi"("SensorADValueIN"=0.0) -> ("SensorADValueOut"=w522:dbl)  [unwired: 3 in, 1 out]
                  n199 = property on="电桥电平" class="DigNum (严格)"("Value"=w522) -> ()  [unwired: 2 in, 2 out]
                  n200 = property on="电桥电平_Event" class="DigNum (严格)"("Value"=w522) -> ()  [unwired: 2 in, 2 out]
                }
                frame "GetSolenStatue" {
                  n201 = Initialize Array(0 ("元素"), 48 ("维数大小")) -> (w525:i32[])
                  n202 = call "API get solen statue.vi"("solenstatue input"=w525) -> ("solenstatue output"=w524:i32[])  [unwired: 10 in]
                  n203 = for {
                    tunnel: w524 -> [w531] mode=indexing
                    i -> [w534]
                    n204 = Not Equal To 0?(x=w531) -> (x != 0?=w532:bool)
                    n205 = Increment(x=w534) -> (x+1=w536:i32)
                    n206 = Number To Decimal String(number=w536) -> (decimal integer string=w535:string)  [unwired: 1 in]
                    n207 = To Variant(anything=w532) -> (Variant=w529:variant)
                    n208 = control-ref of="本VI"() -> (w530:refnum<vi>)
                    n209 = Concatenate Strings("Solen" ("字符串"), w535) -> (w528:string)
                    n210 = invoke class="VI" method="Ctrl Val.Set"(reference=w530, "Control Name"=w528, "Value"=w529) -> ()  [unwired: 2 in, 5 out]
                  }
                }
                frame "GetPaltformStatue" {
                  n211 = Initialize Array(0 ("元素"), 8 ("维数大小")) -> (w548:i32[])
                  n212 = Initialize Array(0 ("元素"), 8 ("维数大小")) -> (w545:i32[])
                  n213 = Initialize Array(0 ("元素"), 8 ("维数大小")) -> (w543:i32[])
                  n214 = call "API get platform statue.vi"("platformStatue input"=w548, "PlatformNum"=1) -> ("platformStatue output"=w537:i32[])  [unwired: 8 in, 1 out]
                  n215 = for {
                    tunnel: w537 -> [w555] mode=indexing
                    i -> [w558]
                    n216 = Not Equal To 0?(x=w555) -> (x != 0?=w556:bool)
                    n217 = To Variant(anything=w556) -> (Variant=w553:variant)
                    n218 = Increment(x=w558) -> (x+1=w560:i32)
                    n219 = Number To Decimal String(number=w560) -> (decimal integer string=w559:string)  [unwired: 1 in]
                    n220 = control-ref of="本VI"() -> (w554:refnum<vi>)
                    n221 = Concatenate Strings("Plat1IO" ("字符串"), w559) -> (w552:string)
                    n222 = invoke class="VI" method="Ctrl Val.Set"(reference=w554, "Control Name"=w552, "Value"=w553) -> ()  [unwired: 2 in, 5 out]
                  }
                  n223 = call "API get platform statue.vi"("platformStatue input"=w545, "PlatformNum"=3) -> ("platformStatue output"=w539:i32[])  [unwired: 8 in, 1 out]
                  n224 = call "API get platform statue.vi"("platformStatue input"=w543, "PlatformNum"=2) -> ("platformStatue output"=w538:i32[])  [unwired: 8 in, 1 out]
                  n225 = for {
                    tunnel: w539 -> [w573] mode=indexing
                    i -> [w576]
                    n226 = Increment(x=w576) -> (x+1=w578:i32)
                    n227 = Not Equal To 0?(x=w573) -> (x != 0?=w574:bool)
                    n228 = Number To Decimal String(number=w578) -> (decimal integer string=w577:string)  [unwired: 1 in]
                    n229 = control-ref of="本VI"() -> (w572:refnum<vi>)
                    n230 = Concatenate Strings("Plat3IO" ("字符串"), w577) -> (w570:string)
                    n231 = To Variant(anything=w574) -> (Variant=w571:variant)
                    n232 = invoke class="VI" method="Ctrl Val.Set"(reference=w572, "Control Name"=w570, "Value"=w571) -> ()  [unwired: 2 in, 5 out]
                  }
                  n233 = for {
                    tunnel: w538 -> [w564] mode=indexing
                    i -> [w567]
                    n234 = Increment(x=w567) -> (x+1=w569:i32)
                    n235 = Not Equal To 0?(x=w564) -> (x != 0?=w565:bool)
                    n236 = Number To Decimal String(number=w569) -> (decimal integer string=w568:string)  [unwired: 1 in]
                    n237 = control-ref of="本VI"() -> (w563:refnum<vi>)
                    n238 = Concatenate Strings("Plat2IO" ("字符串"), w568) -> (w561:string)
                    n239 = To Variant(anything=w565) -> (Variant=w562:variant)
                    n240 = invoke class="VI" method="Ctrl Val.Set"(reference=w563, "Control Name"=w561, "Value"=w562) -> ()  [unwired: 2 in, 5 out]
                  }
                }
                frame "GetMotorStatue" {
                  n241 = Initialize Array(0 ("元素"), 6 ("维数大小")) -> (w582:i32[])
                  n242 = call "API get motor statue.vi"("motor statue array input"=w582) -> ("motor statue array output"=w579:i32[])  [unwired: 9 in, 1 out]
                  n243 = for {
                    tunnel: w579 -> [w586] mode=indexing
                    i -> [w589]
                    n244 = Not Equal To 0?(x=w586) -> (x != 0?=w587:bool)
                    n245 = Increment(x=w589) -> (x+1=w591:i32)
                    n246 = Number To Decimal String(number=w591) -> (decimal integer string=w590:string)  [unwired: 1 in]
                    n247 = To Variant(anything=w587) -> (Variant=w584:variant)
                    n248 = control-ref of="本VI"() -> (w585:refnum<vi>)
                    n249 = Concatenate Strings("M" ("字符串"), w590) -> (w583:string)
                    n250 = invoke class="VI" method="Ctrl Val.Set"(reference=w585, "Control Name"=w583, "Value"=w584) -> ()  [unwired: 2 in, 5 out]
                  }
                }
                frame "FeedMotorStart" {
                  n251 = call "API Feed Motor START.vi"() -> ()  [unwired: 11 in, 1 out]
                }
                frame "FeedMotorStop" {
                  n252 = call "API Feed Motor Stop.vi"() -> ()  [unwired: 11 in, 1 out]
                }
                frame "MotorStart" {
                  n253 = Dequeue Element(queue=w594, error in (no error)=w593) -> (element=w592:i32)  [unwired: 1 in, 3 out]
                  n254 = Dequeue Element(queue=w600, error in (no error)=w599) -> (element=w598:i32)  [unwired: 1 in, 3 out]
                  n255 = Dequeue Element(queue=w597, error in (no error)=w596) -> (element=w595:i32)  [unwired: 1 in, 3 out]
                  n256 = call "API Motor Start.vi"("stepNum"=w598, "direction"=w595, "motorNum"=w592) -> ()  [unwired: 8 in, 1 out]
                }
                frame "MotorRestart" {
                }
                frame "MotorStop" {
                  n257 = call "API Motor Stop.vi"() -> ()  [unwired: 11 in, 1 out]
                }
                frame "SolenAction" {
                  n258 = Dequeue Element(queue=w604, error in (no error)=w603) -> (element=w601:i32)  [unwired: 1 in, 3 out]
                  n259 = Dequeue Element(queue=w606, error in (no error)=w605) -> (element=w602:i32)  [unwired: 1 in, 3 out]
                  n260 = call "API Solen Action.vi"("statue"=w601, "solenNum"=w602) -> ()  [unwired: 9 in, 1 out]
                }
                frame "SolenAdv" {
                  n261 = Dequeue Element(queue=w612, error in (no error)=w611) -> (element=w608:i32)  [unwired: 1 in, 3 out]
                  n262 = Dequeue Element(queue=w610, error in (no error)=w609) -> (element=w607:i32)  [unwired: 1 in, 3 out]
                  n263 = call "API Solen Advance.vi"("statue"=w607, "platformNum"=w608) -> ()  [unwired: 9 in, 1 out]
                }
                frame "RcvDataInit" {
                  n264 = call "API Rcv Data Init.vi"() -> ()  [unwired: 2 in, 2 out]
                }
                frame "SetMotorSpeed" {
                  n265 = Dequeue Element(queue=w618, error in (no error)=w617) -> (element=w614:i32)  [unwired: 1 in, 3 out]
                  n266 = Dequeue Element(queue=w616, error in (no error)=w615) -> (element=w613:i32)  [unwired: 1 in, 3 out]
                  n267 = call "API Set Motor Speed.vi"("motorSpeed"=w613, "motorNum"=w614) -> ()  [unwired: 9 in, 1 out]
                }
              }
              n268 = Get Queue Status(queue=w500, error in (no error)=w499) -> (# elements in queue=w482:i32)  [unwired: 1 in, 7 out]
              "指令数" <- w482
              n269 = local read "stop"() -> (w497:bool)
              n270 = And(x=w497, y=TRUE) -> (x .and. y?=w481:bool)
              n271 = Equal To 0?(x=w482) -> (x = 0?=w480:bool)
              n272 = And(x=w481, y=w480) -> (x .and. y?=w479:bool)
            }
            frame Error {
            }
          }
        }
      }
    }
  }
  n273 = while {
    tunnel: w220 -> [_]
    tunnel: w218 -> [_]
    tunnel: w216 -> [_]
    tunnel: w215 -> [_]
    tunnel: w214 -> [_]
    tunnel: w206 -> [_]
    tunnel: w205 -> [_]
    tunnel: w202 -> [_]
    tunnel: w200 -> [_]
    tunnel: w172 -> [w622]
    tunnel: w171 -> [w621]
    tunnel: w196 -> [_]
    tunnel: w187 -> [_]
    tunnel: w186 -> [_]
    tunnel: w184 -> [_]
    tunnel: w183 -> [_]
    tunnel: w180 -> [_]
    tunnel: w178 -> [_]
    tunnel: "选项卡控件" -> [_]
    tunnel: "选项卡控件Next" -> [_]
    stop <- FALSE stop-if-true
    n274 = event shown="[1] \"start\": 值改变" {
      selector: _ -> [_ _ _]
      dyn-events: _ -> [_ _ _]
      timeout: _ -> [_ _ _]
      tunnel: w622 -> [_ w626 w729]
      tunnel: w621 -> [_ w625 w728]
      event Timeout {
        n275 = event-data() -> ()  [unwired: 1 in, 2 out]
      }
      event "start": Value Change {
        n276 = event-data() -> ()  [unwired: 1 in, 5 out]
        n277 = Flush Queue(queue=w626, error in (no error)=w625) -> (queue out=w624:refnum<queue>, error out=w623:errorcluster)  [unwired: 1 out]
        n278 = call "API SYSINIT.vi"() -> ("SYSINIT return value"=w627:bool)  [unwired: 11 in]
        n279 = property on="Statue" class="Bool (严格)"("Value"=w627) -> ()  [unwired: 2 in, 2 out]
        n280 = case shown="真" w627 {
          tunnel: w624 -> [_ w637]
          tunnel: w623 -> [_ w636]
          frame False {
          }
          frame True {
            w630 = T2."Enabled" ("禁用")
            w641 = T2."Enabled" ("禁用")
            n281 = node-c288() -> (w629:T6)  [unwired: 4 in]
            n282 = timed-loop {
              shift-right: [w652] -> _
              shift-left: w637 -> [w660]
              shift-right: [w651] -> _
              shift-left: w636 -> [w659]
              timing: w629 -> [_]
              timing-out: [_] -> w628
              stop <- w648 stop-if-true
              n283 = node-c288() -> ()  [unwired: 1 in, 1 out]
              n284 = local read "stop"() -> (w649:bool)
              n285 = And(x=w649, y=TRUE) -> (x .and. y?=w648:bool)
              n286 = Enqueue Element(queue=w660, element=T5."RcvDataInit" ("元素"), error in (no error)=w659) -> (queue out=w662:refnum<queue>, error out=w661:errorcluster)  [unwired: 1 in, 1 out]
              n287 = Enqueue Element(queue=w662, element=T5."GetSensorStatue" ("元素"), error in (no error)=w661) -> (queue out=w670:refnum<queue>, error out=w669:errorcluster)  [unwired: 1 in, 1 out]
              n288 = Enqueue Element(queue=w670, element=T5."GetSensorAD" ("元素"), error in (no error)=w669) -> (queue out=w668:refnum<queue>, error out=w667:errorcluster)  [unwired: 1 in, 1 out]
              n289 = Enqueue Element(queue=w668, element=T5."GetSolenStatue" ("元素"), error in (no error)=w667) -> (queue out=w666:refnum<queue>, error out=w665:errorcluster)  [unwired: 1 in, 1 out]
              n290 = Enqueue Element(queue=w666, element=T5."GetPaltformStatue" ("元素"), error in (no error)=w665) -> (queue out=w664:refnum<queue>, error out=w663:errorcluster)  [unwired: 1 in, 1 out]
              n291 = Enqueue Element(queue=w664, element=T5."GetMotorStatue" ("元素"), error in (no error)=w663) -> (queue out=w652:refnum<queue>, error out=w651:errorcluster)  [unwired: 1 in, 1 out]
              n292 = node-c288() -> ()  [unwired: 1 in, 1 out]
            }
            n293 = while {
              shift-right: [w688] -> _
              shift-left: 0 -> [w690]
              shift-right: [w689] -> _
              shift-left: enum16{"允许计数", "不允许计数"}."允许计数" -> [w691]
              shift-right: [w682] -> _
              shift-left: enum16{"允许计数", "不允许计数"}."允许计数" -> [w684]
              shift-right: [w681] -> _
              shift-left: 0 -> [w683]
              stop <- w685 stop-if-true
              n294 = local read "stop"() -> (w687:bool)
              n295 = Wait (ms)(milliseconds to wait=u32 10 ("等待时间（毫秒）")) -> ()  [unwired: 1 out]
              n296 = And(x=w687, y=TRUE) -> (x .and. y?=w685:bool)
              n297 = property on="电桥电平_Event" class="DigNum (严格)"() -> ("Value"=w679:dbl)  [unwired: 2 in, 2 out]
              n298 = property on="KCurrent" class="DigNum (严格)"() -> ("Value"=w678:dbl)  [unwired: 2 in, 2 out]
              n299 = property on="BCurrent" class="DigNum (严格)"() -> ("Value"=w676:dbl)  [unwired: 2 in, 2 out]
              n300 = case shown="\"允许计数\", 默认" w684 {
                tunnel: w683 -> [w694 w703]
                tunnel: [w693 w703] -> w681
                tunnel: [w692 w704] -> w682
                frame "允许计数", Default {
                  n301 = property on="红外电平" class="DigNum (严格)"() -> ("Value"=w697:dbl)  [unwired: 2 in, 2 out]
                  n302 = Greater?(x=w697, y=0.5) -> (0:w695:bool)
                  n303 = case shown="假" w695 {
                    tunnel: w694 -> [w698 w702]
                    tunnel: [w698 w701] -> w693
                    tunnel: [enum16{"允许计数", "不允许计数"}."允许计数" enum16{"允许计数", "不允许计数"}."不允许计数"] -> w692
                    frame False {
                    }
                    frame True {
                      n304 = Increment(x=w702) -> (x+1=w701:i32)
                    }
                  }
                }
                frame "不允许计数" {
                  n305 = property on="红外电平" class="DigNum (严格)"() -> ("Value"=w707:dbl)  [unwired: 2 in, 2 out]
                  n306 = Less?(x=w707, y=0.5) -> (x < y?=w705:bool)
                  n307 = case shown="假" w705 {
                    tunnel: [enum16{"允许计数", "不允许计数"}."不允许计数" enum16{"允许计数", "不允许计数"}."允许计数"] -> w704
                    frame False {
                    }
                    frame True {
                    }
                  }
                }
              }
              n308 = case shown="\"允许计数\", 默认" w691 {
                tunnel: w690 -> [w712 w721]
                tunnel: [w711 w721] -> w688
                tunnel: [w710 w722] -> w689
                frame "允许计数", Default {
                  n309 = property on="电涡流电平" class="DigNum (严格)"() -> ("Value"=w715:dbl)  [unwired: 2 in, 2 out]
                  n310 = Greater?(x=w715, y=0.5) -> (0:w713:bool)
                  n311 = case shown="假" w713 {
                    tunnel: w712 -> [w716 w720]
                    tunnel: [w716 w719] -> w711
                    tunnel: [enum16{"允许计数", "不允许计数"}."允许计数" enum16{"允许计数", "不允许计数"}."不允许计数"] -> w710
                    frame False {
                    }
                    frame True {
                      n312 = Increment(x=w720) -> (x+1=w719:i32)
                    }
                  }
                }
                frame "不允许计数" {
                  n313 = property on="电涡流电平" class="DigNum (严格)"() -> ("Value"=w725:dbl)  [unwired: 2 in, 2 out]
                  n314 = Less?(x=w725, y=0.5) -> (x < y?=w723:bool)
                  n315 = case shown="假" w723 {
                    tunnel: [enum16{"允许计数", "不允许计数"}."不允许计数" enum16{"允许计数", "不允许计数"}."允许计数"] -> w722
                    frame False {
                    }
                    frame True {
                    }
                  }
                }
              }
              n316 = Multiply(x=w679, y=w678) -> (x*y=w677:dbl)
              n317 = Add(x=w677, y=w676) -> (x+y=w675:dbl)
              n318 = property on="Stog" class="DigNum (严格)"("Value"=w675) -> ()  [unwired: 2 in, 2 out]
              n319 = property on="红外计数" class="DigNum (严格)"("Value"=w681) -> ()  [unwired: 2 in, 2 out]
              n320 = property on="电涡流计数" class="DigNum (严格)"("Value"=w688) -> ()  [unwired: 2 in, 2 out]
            }
            n321 = property on="stop" class="Bool (严格)"("DisabledEnum"=w641) -> (error out=w640:errorcluster)  [unwired: 2 in, 1 out]
            n322 = property on="restartbtn" class="Bool"(error in=w640, "DisabledEnum"=w641) -> (error out=w639:errorcluster)  [unwired: 1 in, 1 out]
            n323 = property on="start" class="Bool"(error in=w639, "DisabledEnum"=T2."Disabled and Grayed Out" ("禁用")) -> (error out=w638:errorcluster)  [unwired: 1 in, 1 out]
            n324 = property on="ClearButton" class="Bool (严格)"(error in=w638, "DisabledEnum"=T2."Disabled and Grayed Out" ("禁用")) -> (error out=w635:errorcluster)  [unwired: 1 in, 1 out]
            n325 = property on="No1Btn" class="Bool"(error in=w635, "DisabledEnum"=w630) -> (error out=w634:errorcluster)  [unwired: 1 in, 1 out]
            n326 = property on="No2Btn" class="Bool"(error in=w634, "DisabledEnum"=w630) -> (error out=w633:errorcluster)  [unwired: 1 in, 1 out]
            n327 = property on="No3Btn" class="Bool"(error in=w633, "DisabledEnum"=w630) -> (error out=w632:errorcluster)  [unwired: 1 in, 1 out]
            n328 = node-c288(w628) -> ()  [unwired: 1 out]
            n329 = property on="BaseBtn" class="Bool"(error in=w632, "DisabledEnum"=w630) -> (error out=w631:errorcluster)  [unwired: 1 in, 1 out]
            n330 = property on="MotinAdv" class="Bool"(error in=w631, "DisabledEnum"=w630) -> ()  [unwired: 1 in, 2 out]
          }
        }
      }
      event "stop": Value Change {
        n331 = event-data() -> ()  [unwired: 1 in, 5 out]
        n332 = flat-sequence {
          tunnel: w729 -> [w731]
          tunnel: w728 -> [w730]
          frame #0 {
            n333 = Flush Queue(queue=w731, error in (no error)=w730) -> ()  [unwired: 3 out]
          }
          frame #1 {
            w732 = T2."Disabled and Grayed Out" ("禁用")
            n334 = property on="start" class="Bool"("DisabledEnum"=T2."Enabled" ("禁用")) -> (error out=w746:errorcluster)  [unwired: 2 in, 1 out]
            n335 = property on="stop" class="Bool (严格)"(error in=w746, "DisabledEnum"=T2."Disabled and Grayed Out" ("禁用")) -> (error out=w743:errorcluster)  [unwired: 1 in, 1 out]
            n336 = property on="stop" class="Bool (严格)"(error in=w743, "Value"=FALSE ("stop")) -> (error out=w742:errorcluster)  [unwired: 1 in, 1 out]
            n337 = property on="ClearButton" class="Bool (严格)"(error in=w742, "DisabledEnum"=T2."Enabled" ("禁用")) -> (error out=w740:errorcluster)  [unwired: 1 in, 1 out]
            n338 = property on="restartbtn" class="Bool"(error in=w740, "DisabledEnum"=w732) -> (error out=w739:errorcluster)  [unwired: 1 in, 1 out]
            n339 = property on="Statue" class="Bool (严格)"(error in=w739, "Value"=FALSE ("Statue")) -> (error out=w737:errorcluster)  [unwired: 1 in, 1 out]
            n340 = property on="No1Btn" class="Bool"(error in=w737, "DisabledEnum"=w732) -> (error out=w736:errorcluster)  [unwired: 1 in, 1 out]
            n341 = property on="No2Btn" class="Bool"(error in=w736, "DisabledEnum"=w732) -> (error out=w735:errorcluster)  [unwired: 1 in, 1 out]
            n342 = property on="No3Btn" class="Bool"(error in=w735, "DisabledEnum"=w732) -> (error out=w734:errorcluster)  [unwired: 1 in, 1 out]
            n343 = property on="BaseBtn" class="Bool"(error in=w734, "DisabledEnum"=w732) -> (error out=w733:errorcluster)  [unwired: 1 in, 1 out]
            n344 = property on="MotinAdv" class="Bool"(error in=w733, "DisabledEnum"=w732) -> ()  [unwired: 1 in, 2 out]
          }
          frame #2 {
            n345 = call "API SYSQUIT.vi"() -> ()  [unwired: 12 in]
          }
        }
      }
    }
  }
  n346 = while {
    tunnel: w171 -> [w764]
    tunnel: w172 -> [w765]
    tunnel: w154 -> [w763]
    tunnel: w153 -> [w762]
    tunnel: w152 -> [w761]
    tunnel: w151 -> [w760]
    tunnel: w150 -> [w759]
    tunnel: w149 -> [w758]
    tunnel: w170 -> [w757]
    tunnel: w168 -> [w756]
    tunnel: w162 -> [w755]
    tunnel: w160 -> [w754]
    tunnel: w169 -> [w753]
    tunnel: w167 -> [w752]
    tunnel: w161 -> [w751]
    tunnel: w159 -> [w750]
    tunnel: w156 -> [w749]
    tunnel: w155 -> [w748]
    stop <- FALSE stop-if-true
    n347 = event shown="[4] \"No3Btn\": 值改变" {
      selector: _ -> [_ _ _ _ _]
      dyn-events: _ -> [_ _ _ _ _]
      timeout: _ -> [_ _ _ _ _]
      tunnel: w765 -> [_ w808 w867 _ w924]
      tunnel: w764 -> [_ _ w866 _ w923]
      tunnel: w763 -> [_ w806 w865 _ w922]
      tunnel: w762 -> [_ w805 w864 _ w921]
      tunnel: w761 -> [_ w802 w863 _ w920]
      tunnel: w760 -> [_ _ w862 _ w919]
      tunnel: w759 -> [_ w801 w861 _ w918]
      tunnel: w758 -> [_ _ w860 _ w917]
      tunnel: w757 -> [_ _ w859 _ _]
      tunnel: w756 -> [_ _ w857 _ _]
      tunnel: w755 -> [_ w798 w855 _ _]
      tunnel: w754 -> [_ w797 w853 _ _]
      tunnel: w753 -> [_ _ w858 _ _]
      tunnel: w752 -> [_ _ w856 _ _]
      tunnel: w751 -> [_ _ w854 _ _]
      tunnel: w750 -> [_ _ w852 _ _]
      tunnel: w749 -> [_ _ _ _ _]
      tunnel: w748 -> [_ _ _ _ _]
      event Timeout {
        n348 = event-data() -> ()  [unwired: 1 in, 2 out]
      }
      event "restartbtn": Value Change {
        n349 = event-data() -> ()  [unwired: 1 in, 5 out]
        n350 = Flush Queue(queue=w806, error in (no error)=w805) -> (queue out=w804:refnum<queue>, error out=w803:errorcluster)  [unwired: 1 out]
        n351 = Enqueue Element(queue=w804, element=20000 ("元素"), error in (no error)=w803) -> (queue out=w844:refnum<queue>, error out=w850:errorcluster)  [unwired: 1 in, 1 out]
        n352 = Flush Queue(queue=w802) -> (queue out=w800:refnum<queue>)  [unwired: 1 in, 2 out]
        n353 = Enqueue Element(queue=w800, element=1 ("元素"), error in (no error)=w850) -> (queue out=w843:refnum<queue>, error out=w849:errorcluster)  [unwired: 1 in, 1 out]
        n354 = Flush Queue(queue=w801) -> (queue out=w799:refnum<queue>)  [unwired: 1 in, 2 out]
        n355 = Enqueue Element(queue=w799, element=3 ("元素"), error in (no error)=w849) -> (queue out=w842:refnum<queue>, error out=w848:errorcluster)  [unwired: 1 in, 1 out]
        n356 = Flush Queue(queue=w808) -> (queue out=w807:refnum<queue>)  [unwired: 1 in, 2 out]
        n357 = Enqueue Element(queue=w807, element=T9."MotorStart" ("元素"), error in (no error)=w848) -> (queue out=w837:refnum<queue>, error out=w841:errorcluster)  [unwired: 1 in, 1 out]
        n358 = Enqueue Element(queue=w844, element=20000 ("元素"), error in (no error)=w841) -> (queue out=w823:refnum<queue>, error out=w840:errorcluster)  [unwired: 1 in, 1 out]
        n359 = Enqueue Element(queue=w843, element=1 ("元素"), error in (no error)=w840) -> (queue out=w821:refnum<queue>, error out=w839:errorcluster)  [unwired: 1 in, 1 out]
        n360 = Enqueue Element(queue=w842, element=4 ("元素"), error in (no error)=w839) -> (queue out=w819:refnum<queue>, error out=w838:errorcluster)  [unwired: 1 in, 1 out]
        n361 = Enqueue Element(queue=w837, element=T9."MotorStart" ("元素"), error in (no error)=w838) -> (queue out=w829:refnum<queue>, error out=w832:errorcluster)  [unwired: 1 in, 1 out]
        n362 = Enqueue Element(queue=w823, element=20000 ("元素"), error in (no error)=w832) -> (queue out=w822:refnum<queue>, error out=w831:errorcluster)  [unwired: 1 in, 1 out]
        n363 = Enqueue Element(queue=w821, element=0 ("元素"), error in (no error)=w831) -> (queue out=w820:refnum<queue>, error out=w830:errorcluster)  [unwired: 1 in, 1 out]
        n364 = Enqueue Element(queue=w819, element=5 ("元素"), error in (no error)=w830) -> (queue out=w818:refnum<queue>, error out=w828:errorcluster)  [unwired: 1 in, 1 out]
        n365 = Enqueue Element(queue=w829, element=T9."MotorStart" ("元素"), error in (no error)=w828) -> (queue out=w817:refnum<queue>, error out=w827:errorcluster)  [unwired: 1 in, 1 out]
        n366 = Enqueue Element(queue=w822, element=20000 ("元素"), error in (no error)=w827) -> (error out=w826:errorcluster)  [unwired: 1 in, 2 out]
        n367 = Enqueue Element(queue=w820, element=1 ("元素"), error in (no error)=w826) -> (error out=w825:errorcluster)  [unwired: 1 in, 2 out]
        n368 = Enqueue Element(queue=w818, element=6 ("元素"), error in (no error)=w825) -> (error out=w824:errorcluster)  [unwired: 1 in, 2 out]
        n369 = Enqueue Element(queue=w817, element=T9."MotorStart" ("元素"), error in (no error)=w824) -> (queue out=w793:refnum<queue>, error out=w796:errorcluster)  [unwired: 1 in, 1 out]
        n370 = Flush Queue(queue=w798) -> (queue out=w791:refnum<queue>)  [unwired: 1 in, 2 out]
        n371 = Enqueue Element(queue=w791, element=0 ("元素"), error in (no error)=w796) -> (queue out=w783:refnum<queue>, error out=w795:errorcluster)  [unwired: 1 in, 1 out]
        n372 = Flush Queue(queue=w797) -> (queue out=w790:refnum<queue>)  [unwired: 1 in, 2 out]
        n373 = Enqueue Element(queue=w790, element=0 ("元素"), error in (no error)=w795) -> (queue out=w782:refnum<queue>, error out=w794:errorcluster)  [unwired: 1 in, 1 out]
        n374 = Enqueue Element(queue=w793, element=T9."SolenAdv" ("元素"), error in (no error)=w794) -> (queue out=w785:refnum<queue>, error out=w787:errorcluster)  [unwired: 1 in, 1 out]
        n375 = Enqueue Element(queue=w783, element=1 ("元素"), error in (no error)=w787) -> (queue out=w774:refnum<queue>, error out=w786:errorcluster)  [unwired: 1 in, 1 out]
        n376 = Enqueue Element(queue=w782, element=0 ("元素"), error in (no error)=w786) -> (queue out=w773:refnum<queue>, error out=w780:errorcluster)  [unwired: 1 in, 1 out]
        n377 = Enqueue Element(queue=w785, element=T9."SolenAdv" ("元素"), error in (no error)=w780) -> (queue out=w778:refnum<queue>, error out=w777:errorcluster)  [unwired: 1 in, 1 out]
        n378 = Enqueue Element(queue=w774, element=2 ("元素"), error in (no error)=w777) -> (error out=w776:errorcluster)  [unwired: 1 in, 2 out]
        n379 = Enqueue Element(queue=w773, element=0 ("元素"), error in (no error)=w776) -> (error out=w775:errorcluster)  [unwired: 1 in, 2 out]
        n380 = Enqueue Element(queue=w778, element=T9."SolenAdv" ("元素"), error in (no error)=w775) -> (queue out=w769:refnum<queue>, error out=w768:errorcluster)  [unwired: 1 in, 1 out]
        n381 = Enqueue Element(queue=w769, element=T9."FeedMotorStop" ("元素"), error in (no error)=w768) -> ()  [unwired: 1 in, 3 out]
      }
      event "No1Btn": Value Change {
        n382 = event-data() -> ()  [unwired: 1 in, 5 out]
        n383 = disable-structure shown="禁用" {
          disable-tunnel: w867 -> [w907 _]
          disable-tunnel: w866 -> [w906 _]
          disable-tunnel: w865 -> [w903 _]
          disable-tunnel: w864 -> [w902 _]
          disable-tunnel: w863 -> [w901 _]
          disable-tunnel: w862 -> [w900 _]
          disable-tunnel: w861 -> [w899 _]
          disable-tunnel: w860 -> [w898 _]
          disable-tunnel: w859 -> [w897 _]
          disable-tunnel: w858 -> [w896 _]
          disable-tunnel: w857 -> [w895 _]
          disable-tunnel: w856 -> [w894 _]
          disable-tunnel: w855 -> [w893 _]
          disable-tunnel: w854 -> [w892 _]
          disable-tunnel: w853 -> [w891 _]
          disable-tunnel: w852 -> [w890 _]
          frame Disabled {
            n384 = Flush Queue(queue=w903, error in (no error)=w902) -> ()  [unwired: 3 out]
            n385 = Flush Queue(queue=w907, error in (no error)=w906) -> (queue out=w905:refnum<queue>, error out=w904:errorcluster)  [unwired: 1 out]
            n386 = Enqueue Element(queue=w905, element=T9."FeedMotorStart" ("元素"), error in (no error)=w904) -> (queue out=w882:refnum<queue>, error out=w889:errorcluster)  [unwired: 1 in, 1 out]
            n387 = Flush Queue(queue=w897, error in (no error)=w896) -> (queue out=w888:refnum<queue>)  [unwired: 2 out]
            n388 = Enqueue Element(queue=w888, element=5 ("元素"), error in (no error)=w889) -> (queue out=w878:refnum<queue>, error out=w886:errorcluster)  [unwired: 1 in, 1 out]
            n389 = Flush Queue(queue=w895, error in (no error)=w894) -> (queue out=w887:refnum<queue>)  [unwired: 2 out]
            n390 = Enqueue Element(queue=w887, element=1 ("元素"), error in (no error)=w886) -> (queue out=w877:refnum<queue>, error out=w883:errorcluster)  [unwired: 1 in, 1 out]
            n391 = Enqueue Element(queue=w882, element=T9."SolenAction" ("元素"), error in (no error)=w883) -> (queue out=w880:refnum<queue>, error out=w879:errorcluster)  [unwired: 1 in, 1 out]
            n392 = while {
              tunnel: w880 -> [w910]
              tunnel: w879 -> [w913]
              tunnel: w878 -> [w912]
              tunnel: w877 -> [w911]
              tunnel: [w913] -> w876
              tunnel: [w912] -> w874
              tunnel: [w911] -> w873
              tunnel: [w910] -> w872
              stop <- w915 stop-if-true
              n393 = property on="红外电平" class="DigNum (严格)"() -> ("Value"=w909:dbl)  [unwired: 2 in, 2 out]
              n394 = Wait (ms)(milliseconds to wait=u32 10 ("等待时间（毫秒）")) -> ()  [unwired: 1 out]
              n395 = Greater?(x=w909, y=0.5) -> (0:w915:bool)
            }
            n396 = Flush Queue(queue=w891, error in (no error)=w890) -> ()  [unwired: 3 out]
            n397 = Flush Queue(queue=w893, error in (no error)=w892) -> ()  [unwired: 3 out]
            n398 = Flush Queue(queue=w899, error in (no error)=w898) -> ()  [unwired: 3 out]
            n399 = Flush Queue(queue=w901, error in (no error)=w900) -> ()  [unwired: 3 out]
            n400 = Enqueue Element(queue=w874, element=5 ("元素"), error in (no error)=w876) -> (error out=w875:errorcluster)  [unwired: 1 in, 2 out]
            n401 = Enqueue Element(queue=w873, element=0 ("元素"), error in (no error)=w875) -> (error out=w871:errorcluster)  [unwired: 1 in, 2 out]
            n402 = Enqueue Element(queue=w872, element=T9."SolenAction" ("元素"), error in (no error)=w871) -> ()  [unwired: 1 in, 3 out]
          }
          frame Enabled {
          }
        }
      }
      event "No2Btn": Value Change {
        n403 = event-data() -> ()  [unwired: 1 in, 5 out]
      }
      event "No3Btn": Value Change {
        n404 = event-data() -> ()  [unwired: 1 in, 5 out]
        n405 = property on="ComboPolicy" class="CmbBox"() -> ("Value"=w925:string)  [unwired: 2 in, 2 out]
        n406 = case shown="\"1\", 默认" w925 {
          tunnel: w924 -> [w959 _]
          tunnel: w923 -> [w958 _]
          tunnel: w922 -> [w957 _]
          tunnel: w921 -> [w946 _]
          tunnel: w920 -> [w956 _]
          tunnel: w919 -> [w955 _]
          tunnel: w918 -> [w954 _]
          tunnel: w917 -> [w953 _]
          frame "1", Default {
            n407 = property on="Horizontal1" class="DigNum (严格)" props=["Value"]() -> ()  [unwired: 2 in, 3 out]
            n408 = property on="Vax1" class="DigNum (严格)" props=["Value"]() -> ()  [unwired: 2 in, 3 out]
            n409 = property on="Vax2" class="DigNum (严格)" props=["Value"]() -> ()  [unwired: 2 in, 3 out]
            n410 = property on="Horizontal2" class="DigNum (严格)" props=["Value"]() -> ()  [unwired: 2 in, 3 out]
            n411 = Flush Queue(queue=w959, error in (no error)=w958) -> (queue out=w948:refnum<queue>)  [unwired: 2 out]
            n412 = Flush Queue(queue=w957, error in (no error)=w946) -> (queue out=w944:refnum<queue>)  [unwired: 2 out]
            n413 = Flush Queue(queue=w956, error in (no error)=w955) -> (queue out=w945:refnum<queue>)  [unwired: 2 out]
            n414 = Flush Queue(queue=w954, error in (no error)=w953) -> (queue out=w952:refnum<queue>, error out=w951:errorcluster)  [unwired: 1 out]
            n415 = Enqueue Element(queue=w952, element=5 ("元素"), error in (no error)=w951) -> (queue out=w936:refnum<queue>, error out=w950:errorcluster)  [unwired: 1 in, 1 out]
            n416 = property on="Horizontal3" class="DigNum (严格)" props=["Value"]() -> ()  [unwired: 2 in, 3 out]
            n417 = property on="Vax3" class="DigNum (严格)" props=["Value"]() -> ()  [unwired: 2 in, 3 out]
            n418 = Enqueue Element(queue=w945, element=0 ("元素"), error in (no error)=w950) -> (queue out=w935:refnum<queue>, error out=w949:errorcluster)  [unwired: 1 in, 1 out]
            n419 = property on="Vax4" class="DigNum (严格)" props=["Value"]() -> ()  [unwired: 2 in, 3 out]
            n420 = property on="Horizontal4" class="DigNum (严格)" props=["Value"]() -> ()  [unwired: 2 in, 3 out]
            n421 = Enqueue Element(queue=w944, element=20000 ("元素"), error in (no error)=w949) -> (queue out=w934:refnum<queue>, error out=w947:errorcluster)  [unwired: 1 in, 1 out]
            n422 = property on="MaxSpeed" class="DigNum (严格)" props=["Value"]() -> ()  [unwired: 2 in, 3 out]
            n423 = property on="MinSpeed" class="DigNum (严格)" props=["Value"]() -> ()  [unwired: 2 in, 3 out]
            n424 = Enqueue Element(queue=w948, element=T3."MotorStart" ("元素"), error in (no error)=w947) -> (queue out=w929:refnum<queue>, error out=w928:errorcluster)  [unwired: 1 in, 1 out]
            n425 = property on="SelectPolicy" class="RadioBtnsControl (严格)" props=["Value"]() -> ()  [unwired: 2 in, 3 out]
            n426 = Enqueue Element(queue=w936, element=6 ("元素"), error in (no error)=w928) -> (error out=w939:errorcluster)  [unwired: 1 in, 2 out]
            n427 = Enqueue Element(queue=w935, element=1 ("元素"), error in (no error)=w939) -> (error out=w938:errorcluster)  [unwired: 1 in, 2 out]
            n428 = Enqueue Element(queue=w934, element=20000 ("元素"), error in (no error)=w938) -> (error out=w937:errorcluster)  [unwired: 1 in, 2 out]
            n429 = Enqueue Element(queue=w929, element=T3."MotorStart" ("元素"), error in (no error)=w937) -> (queue out=w927:refnum<queue>, error out=w926:errorcluster)  [unwired: 1 in, 1 out]
            n430 = flat-sequence {
              tunnel: [w962] -> _
              tunnel: w927 -> [w962]
              tunnel: [w961] -> _
              tunnel: w926 -> [w961]
              frame #0 {
                n431 = Wait (ms)(milliseconds to wait=u32 100 ("等待时间（毫秒）")) -> ()  [unwired: 1 out]
              }
            }
            n432 = property on="M5" class="Bool (严格)" props=["Value"]() -> ()  [unwired: 2 in, 3 out]
            n433 = property on="M6" class="Bool (严格)" props=["Value"]() -> ()  [unwired: 2 in, 3 out]
          }
          frame "2" {
          }
        }
      }
    }
  }
  n434 = while {
    tunnel: w176 -> [_]
    tunnel: w172 -> [w984]
    tunnel: w171 -> [w983]
    tunnel: w170 -> [w982]
    tunnel: w169 -> [w981]
    tunnel: w168 -> [w980]
    tunnel: w167 -> [w979]
    tunnel: w162 -> [w978]
    tunnel: w161 -> [w977]
    tunnel: w160 -> [w976]
    tunnel: w159 -> [w975]
    tunnel: w156 -> [w974]
    tunnel: w155 -> [w973]
    tunnel: w154 -> [w972]
    tunnel: w153 -> [w971]
    tunnel: w152 -> [w970]
    tunnel: w151 -> [w969]
    tunnel: w150 -> [w968]
    tunnel: w149 -> [w967]
    tunnel: w134 -> [_]
    tunnel: "MotorSpeedNum" -> [_]
    tunnel: "MotorSpeed" -> [_]
    tunnel: w47 -> [_]
    tunnel: w38 -> [w966]
    tunnel: w37 -> [w965]
    tunnel: w36 -> [w964]
    tunnel: w35 -> [w963]
    stop <- FALSE stop-if-true
    n435 = event shown="[13] \"SetMotorSpeed\": 值改变" {
      selector: _ -> [_ _ _ _ _ _ _ _ _ _ _ _ _ _]
      dyn-events: _ -> [_ _ _ _ _ _ _ _ _ _ _ _ _ _]
      timeout: _ -> [_ _ _ _ _ _ _ _ _ _ _ _ _ _]
      tunnel: w984 -> [_ w1001 w1028 w1051 w1068 w1077 w1082 _ _ _ _ _ _ w1103]
      tunnel: w983 -> [_ w1000 w1027 w1050 w1067 w1076 w1081 _ _ _ _ _ _ w1102]
      tunnel: w982 -> [_ w999 _ _ _ _ _ _ _ _ _ _ _ _]
      tunnel: w981 -> [_ w998 _ _ _ _ _ _ _ _ _ _ _ _]
      tunnel: w980 -> [_ w997 _ _ _ _ _ _ _ _ _ _ _ _]
      tunnel: w979 -> [_ w996 _ _ _ _ _ _ _ _ _ _ _ _]
      tunnel: w978 -> [_ _ _ _ w1072 _ _ _ _ _ _ _ _ _]
      tunnel: w977 -> [_ _ _ _ w1071 _ _ _ _ _ _ _ _ _]
      tunnel: w976 -> [_ _ _ _ w1070 _ _ _ _ _ _ _ _ _]
      tunnel: w975 -> [_ _ _ _ w1069 _ _ _ _ _ _ _ _ _]
      tunnel: w974 -> [_ _ _ w1056 _ _ _ _ _ _ _ _ _ _]
      tunnel: w973 -> [_ _ _ w1055 _ _ _ _ _ _ _ _ _ _]
      tunnel: w972 -> [_ _ w1026 _ _ _ _ _ _ _ _ _ _ _]
      tunnel: w971 -> [_ _ w1025 _ _ _ _ _ _ _ _ _ _ _]
      tunnel: w970 -> [_ _ w1024 _ _ _ _ _ _ _ _ _ _ _]
      tunnel: w969 -> [_ _ w1023 _ _ _ _ _ _ _ _ _ _ _]
      tunnel: w968 -> [_ _ w1022 _ _ _ _ _ _ _ _ _ _ _]
      tunnel: w967 -> [_ _ w1021 _ _ _ _ _ _ _ _ _ _ _]
      tunnel: w966 -> [_ _ _ _ _ _ _ _ _ _ _ _ _ w1101]
      tunnel: w965 -> [_ _ _ _ _ _ _ _ _ _ _ _ _ w1100]
      tunnel: w964 -> [_ _ _ _ _ _ _ _ _ _ _ _ _ w1099]
      tunnel: w963 -> [_ _ _ _ _ _ _ _ _ _ _ _ _ w1098]
      event Timeout {
        n436 = event-data() -> ()  [unwired: 1 in, 2 out]
      }
      event "SolenAction": Value Change {
        n437 = event-data() -> ()  [unwired: 1 in, 5 out]
        n438 = property on="SolenStatue_Event" class="CmbBox"() -> ("Value"=w989:string)  [unwired: 2 in, 2 out]
        n439 = Decimal String To Number(string=w989) -> (number=w988:i32)  [unwired: 2 in, 1 out]
        n440 = Flush Queue(queue=w997, error in (no error)=w996) -> (queue out=w990:refnum<queue>, error out=w995:errorcluster)  [unwired: 1 out]
        n441 = Enqueue Element(queue=w990, element=w988, error in (no error)=w995) -> (error out=w994:errorcluster)  [unwired: 1 in, 2 out]
        n442 = property on="SolenNum_Event" class="DigNum (严格)"() -> ("Value"=w987:i32)  [unwired: 2 in, 2 out]
        n443 = Flush Queue(queue=w999, error in (no error)=w998) -> (queue out=w991:refnum<queue>)  [unwired: 2 out]
        n444 = Flush Queue(queue=w1001, error in (no error)=w1000) -> (queue out=w992:refnum<queue>)  [unwired: 2 out]
        n445 = Enqueue Element(queue=w991, element=w987, error in (no error)=w994) -> (error out=w993:errorcluster)  [unwired: 1 in, 2 out]
        n446 = Enqueue Element(queue=w992, element=T9."SolenAction" ("元素"), error in (no error)=w993) -> ()  [unwired: 1 in, 3 out]
      }
      event "MotorStart": Value Change {
        n447 = event-data() -> ()  [unwired: 1 in, 5 out]
        n448 = property on="Directon" class="CmbBox"() -> ("Value"=w1012:string)  [unwired: 2 in, 2 out]
        n449 = property on="MotorNum" class="DigNum (严格)"() -> ("Value"=w1009:i32)  [unwired: 2 in, 2 out]
        n450 = Flush Queue(queue=w1022, error in (no error)=w1021) -> (queue out=w1015:refnum<queue>, error out=w1020:errorcluster)  [unwired: 1 out]
        n451 = Flush Queue(queue=w1024, error in (no error)=w1023) -> (queue out=w1016:refnum<queue>)  [unwired: 2 out]
        n452 = Decimal String To Number(string=w1012) -> (number=w1011:i32)  [unwired: 2 in, 1 out]
        n453 = Enqueue Element(queue=w1015, element=w1009, error in (no error)=w1020) -> (error out=w1019:errorcluster)  [unwired: 1 in, 2 out]
        n454 = Enqueue Element(queue=w1016, element=w1011, error in (no error)=w1019) -> (error out=w1018:errorcluster)  [unwired: 1 in, 2 out]
        n455 = property on="StepNum" class="DigNum (严格)"() -> ("Value"=w1008:i32)  [unwired: 2 in, 2 out]
        n456 = Flush Queue(queue=w1026, error in (no error)=w1025) -> (queue out=w1017:refnum<queue>)  [unwired: 2 out]
        n457 = Enqueue Element(queue=w1017, element=w1008, error in (no error)=w1018) -> (error out=w1014:errorcluster)  [unwired: 1 in, 2 out]
        n458 = Flush Queue(queue=w1028, error in (no error)=w1027) -> (queue out=w1013:refnum<queue>)  [unwired: 2 out]
        n459 = property on="Motor4Pos" class="DigNum (严格)"() -> ("Value"=w1004:i32)  [unwired: 2 in, 2 out]
        n460 = property on="Motor5Pos" class="DigNum (严格)"() -> ("Value"=w1003:i32)  [unwired: 2 in, 2 out]
        n461 = property on="Motor6Pos" class="DigNum (严格)"() -> ("Value"=w1002:i32)  [unwired: 2 in, 2 out]
        n462 = Enqueue Element(queue=w1013, element=T9."MotorStart" ("元素"), error in (no error)=w1014) -> ()  [unwired: 1 in, 3 out]
        n463 = property on="Motor1Pos" class="DigNum (严格)"() -> ("Value"=w1007:i32)  [unwired: 2 in, 2 out]
        n464 = property on="Motor2Pos" class="DigNum (严格)"() -> ("Value"=w1006:i32)  [unwired: 2 in, 2 out]
        n465 = property on="Motor3Pos" class="DigNum (严格)"() -> ("Value"=w1005:i32)  [unwired: 2 in, 2 out]
        n466 = case shown="6" w1009 {
          tunnel: w1008 -> [w1029 w1033 w1037 w1040 w1043 w1046]
          tunnel: w1007 -> [w1031 _ _ _ _ _]
          tunnel: w1006 -> [_ w1034 _ _ _ _]
          tunnel: w1005 -> [_ _ w1036 _ _ _]
          tunnel: w1004 -> [_ _ _ w1039 _ _]
          tunnel: w1003 -> [_ _ _ _ w1042 _]
          tunnel: w1002 -> [_ _ _ _ _ w1045]
          frame 1, Default {
            n467 = Add(x=w1029, y=w1031) -> (x+y=w1030:i32)
            n468 = property on="Motor1Pos" class="DigNum (严格)"("Value"=w1030) -> ()  [unwired: 2 in, 2 out]
          }
          frame 2 {
            n469 = Add(x=w1033, y=w1034) -> (x+y=w1032:i32)
            n470 = property on="Motor2Pos" class="DigNum (严格)"("Value"=w1032) -> ()  [unwired: 2 in, 2 out]
          }
          frame 3 {
            n471 = Add(x=w1037, y=w1036) -> (x+y=w1035:i32)
            n472 = property on="Motor3Pos" class="DigNum (严格)"("Value"=w1035) -> ()  [unwired: 2 in, 2 out]
          }
          frame 4 {
            n473 = Add(x=w1040, y=w1039) -> (x+y=w1038:i32)
            n474 = property on="Motor4Pos" class="DigNum (严格)"("Value"=w1038) -> ()  [unwired: 2 in, 2 out]
          }
          frame 5 {
            n475 = Add(x=w1043, y=w1042) -> (x+y=w1041:i32)
            n476 = property on="Motor5Pos" class="DigNum (严格)"("Value"=w1041) -> ()  [unwired: 2 in, 2 out]
          }
          frame 6 {
            n477 = Add(x=w1046, y=w1045) -> (x+y=w1044:i32)
            n478 = property on="Motor6Pos" class="DigNum (严格)"("Value"=w1044) -> ()  [unwired: 2 in, 2 out]
          }
        }
      }
      event "MotorStop": Value Change {
        n479 = event-data() -> ()  [unwired: 1 in, 5 out]
        n480 = Flush Queue(queue=w1056, error in (no error)=w1055) -> (queue out=w1054:refnum<queue>, error out=w1053:errorcluster)  [unwired: 1 out]
        n481 = property on="StopMotorNum" class="DigNum (严格)"() -> ("Value"=w1052:i32)  [unwired: 2 in, 2 out]
        n482 = Flush Queue(queue=w1051, error in (no error)=w1050) -> (queue out=w1049:refnum<queue>)  [unwired: 2 out]
        n483 = Enqueue Element(queue=w1054, element=w1052, error in (no error)=w1053) -> (error out=w1048:errorcluster)  [unwired: 1 in, 2 out]
        n484 = Enqueue Element(queue=w1049, element=T9."MotorStop" ("元素"), error in (no error)=w1048) -> ()  [unwired: 1 in, 3 out]
      }
      event "SolenAdvance": Value Change {
        n485 = event-data() -> ()  [unwired: 1 in, 5 out]
        n486 = property on="SolenPlatStatue_Event" class="CmbBox"() -> ("Value"=w1059:string)  [unwired: 2 in, 2 out]
        n487 = Decimal String To Number(string=w1059) -> (number=w1058:i32)  [unwired: 2 in, 1 out]
        n488 = Flush Queue(queue=w1070, error in (no error)=w1069) -> (queue out=w1061:refnum<queue>, error out=w1066:errorcluster)  [unwired: 1 out]
        n489 = property on="SolenPlat_Event" class="DigNum (严格)"() -> ("Value"=w1060:i32)  [unwired: 2 in, 2 out]
        n490 = Flush Queue(queue=w1072, error in (no error)=w1071) -> (queue out=w1062:refnum<queue>)  [unwired: 2 out]
        n491 = Enqueue Element(queue=w1061, element=w1058, error in (no error)=w1066) -> (error out=w1065:errorcluster)  [unwired: 1 in, 2 out]
        n492 = Enqueue Element(queue=w1062, element=w1060, error in (no error)=w1065) -> (error out=w1064:errorcluster)  [unwired: 1 in, 2 out]
        n493 = Flush Queue(queue=w1068, error in (no error)=w1067) -> (queue out=w1063:refnum<queue>)  [unwired: 2 out]
        n494 = Enqueue Element(queue=w1063, element=T9."SolenAdv" ("元素"), error in (no error)=w1064) -> ()  [unwired: 1 in, 3 out]
      }
      event "FeedMotorStart": Value Change {
        n495 = event-data() -> ()  [unwired: 1 in, 5 out]
        n496 = Flush Queue(queue=w1077, error in (no error)=w1076) -> (queue out=w1075:refnum<queue>, error out=w1074:errorcluster)  [unwired: 1 out]
        n497 = Enqueue Element(queue=w1075, element=T9."FeedMotorStart" ("元素"), error in (no error)=w1074) -> ()  [unwired: 1 in, 3 out]
      }
      event "FeedMotorStop": Value Change {
        n498 = event-data() -> ()  [unwired: 1 in, 5 out]
        n499 = Flush Queue(queue=w1082, error in (no error)=w1081) -> (queue out=w1080:refnum<queue>, error out=w1079:errorcluster)  [unwired: 1 out]
        n500 = Enqueue Element(queue=w1080, element=T9."FeedMotorStop" ("元素"), error in (no error)=w1079) -> ()  [unwired: 1 in, 3 out]
      }
      event "ClearPos1": Value Change {
        n501 = event-data() -> ()  [unwired: 1 in, 5 out]
        n502 = property on="Motor1Pos" class="DigNum (严格)"("Value"=0 ("Motor1Pos")) -> ()  [unwired: 2 in, 2 out]
      }
      event "ClearPos2": Value Change {
        n503 = event-data() -> ()  [unwired: 1 in, 5 out]
        n504 = property on="Motor2Pos" class="DigNum (严格)"("Value"=0 ("Motor2Pos")) -> ()  [unwired: 2 in, 2 out]
      }
      event "ClearPos3": Value Change {
        n505 = event-data() -> ()  [unwired: 1 in, 5 out]
        n506 = property on="Motor3Pos" class="DigNum (严格)"("Value"=0 ("Motor3Pos")) -> ()  [unwired: 2 in, 2 out]
      }
      event "ClearPos4": Value Change {
        n507 = event-data() -> ()  [unwired: 1 in, 5 out]
        n508 = property on="Motor4Pos" class="DigNum (严格)"("Value"=0 ("Motor4Pos")) -> ()  [unwired: 2 in, 2 out]
      }
      event "ClearPos5": Value Change {
        n509 = event-data() -> ()  [unwired: 1 in, 5 out]
        n510 = property on="Motor5Pos" class="DigNum (严格)"("Value"=0 ("Motor5Pos")) -> ()  [unwired: 2 in, 2 out]
      }
      event "ClearPos6": Value Change {
        n511 = event-data() -> ()  [unwired: 1 in, 5 out]
        n512 = property on="Motor6Pos" class="DigNum (严格)"("Value"=0 ("Motor6Pos")) -> ()  [unwired: 2 in, 2 out]
      }
      event "SetMotorSpeed": Value Change {
        n513 = event-data() -> ()  [unwired: 1 in, 5 out]
        n514 = property on="MotorSpeedNum" class="DigNum (严格)"() -> ("Value"=w1091:i32)  [unwired: 2 in, 2 out]
        n515 = Flush Queue(queue=w1101, error in (no error)=w1100) -> (queue out=w1097:refnum<queue>, error out=w1096:errorcluster)  [unwired: 1 out]
        n516 = property on="MotorSpeed" class="DigNum (严格)"() -> ("Value"=w1090:i32)  [unwired: 2 in, 2 out]
        n517 = Flush Queue(queue=w1099, error in (no error)=w1098) -> (queue out=w1095:refnum<queue>)  [unwired: 2 out]
        n518 = Enqueue Element(queue=w1097, element=w1091, error in (no error)=w1096) -> (error out=w1094:errorcluster)  [unwired: 1 in, 2 out]
        n519 = Flush Queue(queue=w1103, error in (no error)=w1102) -> (queue out=w1093:refnum<queue>)  [unwired: 2 out]
        n520 = Enqueue Element(queue=w1095, element=w1090, error in (no error)=w1094) -> (error out=w1092:errorcluster)  [unwired: 1 in, 2 out]
        n521 = Enqueue Element(queue=w1093, element=T3."SetMotorSpeed" ("元素"), error in (no error)=w1092) -> ()  [unwired: 1 in, 3 out]
      }
    }
  }
  n522 = while {
    stop <- FALSE stop-if-true
    n523 = event shown="[3] \"no1btn\": 值改变" {
      selector: _ -> [_ _ _ _ _ _ _ _]
      dyn-events: _ -> [_ _ _ _ _ _ _ _]
      timeout: _ -> [_ _ _ _ _ _ _ _]
      event Timeout {
        n524 = event-data() -> ()  [unwired: 1 in, 2 out]
      }
      event "ClearButton": Value Change {
        n525 = event-data() -> ()  [unwired: 1 in, 5 out]
        n526 = property on="Waveform Chart" class="WFChart (严格)"("History Data"=dynamicdata[] [] ("历史数据")) -> ()  [unwired: 2 in, 2 out]
      }
      event "statuebtn": Value Change {
        n527 = event-data() -> ()  [unwired: 1 in, 5 out]
        n528 = property on="选项卡控件" class="TabCtl (严格)"("Value"=T1."选项卡 2" ("选项卡控件")) -> ()  [unwired: 2 in, 2 out]
      }
      event "no1btn": Value Change {
        n529 = event-data() -> ()  [unwired: 1 in, 5 out]
        n530 = property on="选项卡控件" class="TabCtl (严格)"("Value"=T1."选项卡 3" ("选项卡控件")) -> ()  [unwired: 2 in, 2 out]
      }
      event "no2btn": Value Change {
        n531 = event-data() -> ()  [unwired: 1 in, 5 out]
        n532 = property on="选项卡控件" class="TabCtl (严格)"("Value"=T1."选项卡 4" ("选项卡控件")) -> ()  [unwired: 2 in, 2 out]
      }
      event "no3btn": Value Change {
        n533 = event-data() -> ()  [unwired: 1 in, 5 out]
        n534 = property on="选项卡控件" class="TabCtl (严格)"("Value"=T1."选项卡 5" ("选项卡控件")) -> ()  [unwired: 2 in, 2 out]
      }
      event "Sensor": Value Change {
        n535 = event-data() -> ()  [unwired: 1 in, 5 out]
        n536 = property on="选项卡控件" class="TabCtl (严格)"("Value"=T1."选项卡 1" ("选项卡控件")) -> ()  [unwired: 2 in, 2 out]
      }
      event "BaseBtn": Value Change {
        n537 = event-data() -> ()  [unwired: 1 in, 5 out]
        n538 = property on="选项卡控件" class="TabCtl (严格)"("Value"=T1."选项卡 6" ("选项卡控件")) -> ()  [unwired: 2 in, 2 out]
      }
    }
  }
